vi "MC_7_12d_JW.vi"() -> ()   [LabVIEW 2011]
uses:
  <vilib>/Utility/file.llb/Read From Spreadsheet File (string).vi
  <vilib>/Utility/inputDevices.llb/keyboardAcquire.vi
  <vilib>/Utility/file.llb/Write To Spreadsheet File (DBL).vi
  <vilib>/Utility/file.llb/Write To Spreadsheet File (string).vi
  <vilib>/regexp/Match Regular Expression.xnode
panel:
  out "Rec: Temp":dbl
  out "Comments":string
  out "Folder Index":dbl caption="Length"
  out "Current \nRecord":string[](array[string])
  out "Transformer \nHeaders":string[](array[string])
  out "Current Device ID":string
  out "Column":string
  out "Row":string
  out "Rec: Concentration":dbl
  out "Rec: Solvent":string
  out "Rec: Method":string
  in  "?":T1(tab)
  out "Rec: Material":string
  in  "Treatment Concentration (mM):":dbl=30.0
  in  "Surface Treatment:":string
  in  "# Drops*:":dbl=inf
  in  "Solution Temp (C):":dbl=55.0
  in  "Relative Humidity (%):":dbl=nan
  in  "Room Temp (F):":dbl=nan
  in  "Time (s):":dbl=80.0
  out "Accel (RPM/s):":dbl
  in  "RPM:":dbl=1000.0
  in  "Wait Time (s):":dbl=10.0
  in  "Sample #:":dbl=1.0
  in  "Fabricator:":string="Jeremy"
  in  "Data File":path
  out "Data Folder":path
  in  "Image Folder":path
  out "Image File":path=path "D:/UserData/Desktop/Jeremy/WFU/Research/Programs/VI mods/Image Not Found.png"
  in  "Ramp (s):":dbl=3.0
  out "Calc: Trap Density-STS":dbl format="%#_4e"
  out "New: Trap Density-STS":dbl format="%#_4e"
  out "Rec: Trap Density-STS":dbl caption="Trap Density-STS" format="%#_3e"
  out "Calc: Trap Density-VT":dbl format="%#_4e"
  out "New: Trap Density-VT":dbl format="%#_4e"
  out "Rec: Trap Density-VT":dbl caption="Trap Density-VT" format="%#_3e"
  out "Calc: Onset V":dbl
  out "New: Onset":dbl
  out "Rec: Onset V":dbl caption="Onset V" format="%#_3g"
  out "Calc: Mobility-Lin":dbl format="%#_4e"
  out "New: Mobility-Lin":dbl format="%#_4e"
  out "Rec: Mobility-Lin":dbl caption="Mobility-Lin" format="%#_3e"
  out "Calc: Mobility-Sat":dbl format="%#_4e"
  out "Rec: Length":dbl caption="Length" format="%#_3g"
  out "Rec: Width":dbl caption="Width" format="%#_4g"
  out "Rec: Dielectric (d)":dbl caption="Dielectric (d)" format="%#_3g"
  out "XY Graph":cluster{dbl[], dbl[]}[](graph)
  in  "NumPts":dbl=5.0
  in  "Cancel Button":bool
  in  "Next Button":bool
  in  "Previous Button":bool
  in  "Up Button":bool
  in  "Down Button":bool
  out "Data Name:":string
  in  "Save Changes?":bool
  in  "New: Dielectric":dbl
  in  "New: Length":dbl
  in  "New: Width":dbl
  out "New: Mobility-Sat":dbl format="%#_4e"
  in  "Slide":dbl(slide) step=1.0 scale=-14.3..2.0 scale format="%#_1p"
  in  "Blank Button":bool
  in  "Zoom":i16(slide)=-3 scale=-5.0..5.0
  out "Image Out 2":T2(plugin-control)
  out "Image Out":T2(plugin-control)
  in  "Magnification":u16(ring) items=["5x", "10x", "20x", "50x", "80x"]
  out "Total Width":dbl
  out "Distances":dbl[](array[numeric])
  in  "Undo Button":bool
  in  "Remove Button":bool
  out "Rec: Mobility-Sat":dbl caption="Mobility-Sat" format="%#_3e"
  out "Index":string
  out "Image Name":string
  in  "Export":bool
  out "Calc: VT":dbl
  out "New: VT":dbl
  in  "Manual":bool
  out "XY Graph 2":cluster{dbl[], dbl[]}[](graph)
  in  "Next Button 2":bool
  in  "Previous Button 2":bool
  in  "Slide 2":dbl(slide) step=1.0 scale=-1.0..82.0 scale format="%#_1p"
  out "Calc: STS":dbl
  out "New: STS":dbl
  in  "NumPts 2":dbl=5.0 caption="NumPts"
  out "Rec: VT":dbl caption="Threshold V" format="%#_3g"
  out "Rec: STS":dbl caption="STS" format="%#_3g"
  out "Rec: On/Off":dbl caption="On/Off" format="%#_3e"
  in  "Save Changes? 2":bool
  in  "Save Changes? 3":bool
  out "Date Recorded":string="Date Recorded" caption="Recorded"
  out "Date Created":string caption="Fabricated"
  out "String":string
  in  "No Image":path=path "D:/UserData/Desktop/Jeremy/WFU/Research/Programs/VI mods/Image Not Found.png"
  in  "Project":path=path "D:/UserData/Desktop/Jeremy/WFU/Research/Programs/Mega Awesome/DeviceData.opj"
  out "Index 2":dbl
  out "Array 8":dbl[](array[numeric])
  out "Array 7":dbl[](array[numeric])
  out "ROI Descriptor out":T3 {"Contours"."Type" items=["No Selection", "Point", "Line", "Rectangle", "Oval", "Polygon", "Freehand Region", "Annulus", "Unused2", "Unused3", "Broken Line", "Freehand Line", "Rotated Rectangle"]}
  out "ROI Descriptor":T3 {"Contours"."Type" items=["No Selection", "Point", "Line", "Rectangle", "Oval", "Polygon", "Freehand Region", "Annulus", "Unused2", "Unused3", "Broken Line", "Freehand Line", "Rotated Rectangle"]}
  out "Numeric 3":dbl
  out "Array 6":dbl[][](array[numeric])
  out "Cluster":T4
  out "Array 5":dbl[](array[numeric])
  out "Array 4":dbl[](array[numeric])
  out "Array 3":dbl[](array[numeric])
  out "Numeric 2":dbl
  out "Numeric":dbl
  out "Array 2":dbl[](array[numeric])
  out "Array":dbl[](array[numeric])
  out "MobVi Index":dbl
  out "Table Control 2":string[][](table)
  out "Table Control":string[][](table)
  in  "Row Start":dbl=20.0
  # "Data Locations"
  # "Data Location"
  # "Image Location"
  # "Sample Properties"
  # "*     Inf = Full coverage\n   NaN = Unknown or Not Applicable"
  # "Recorded"
  # "Calculated"
  # "Re-Calculated"
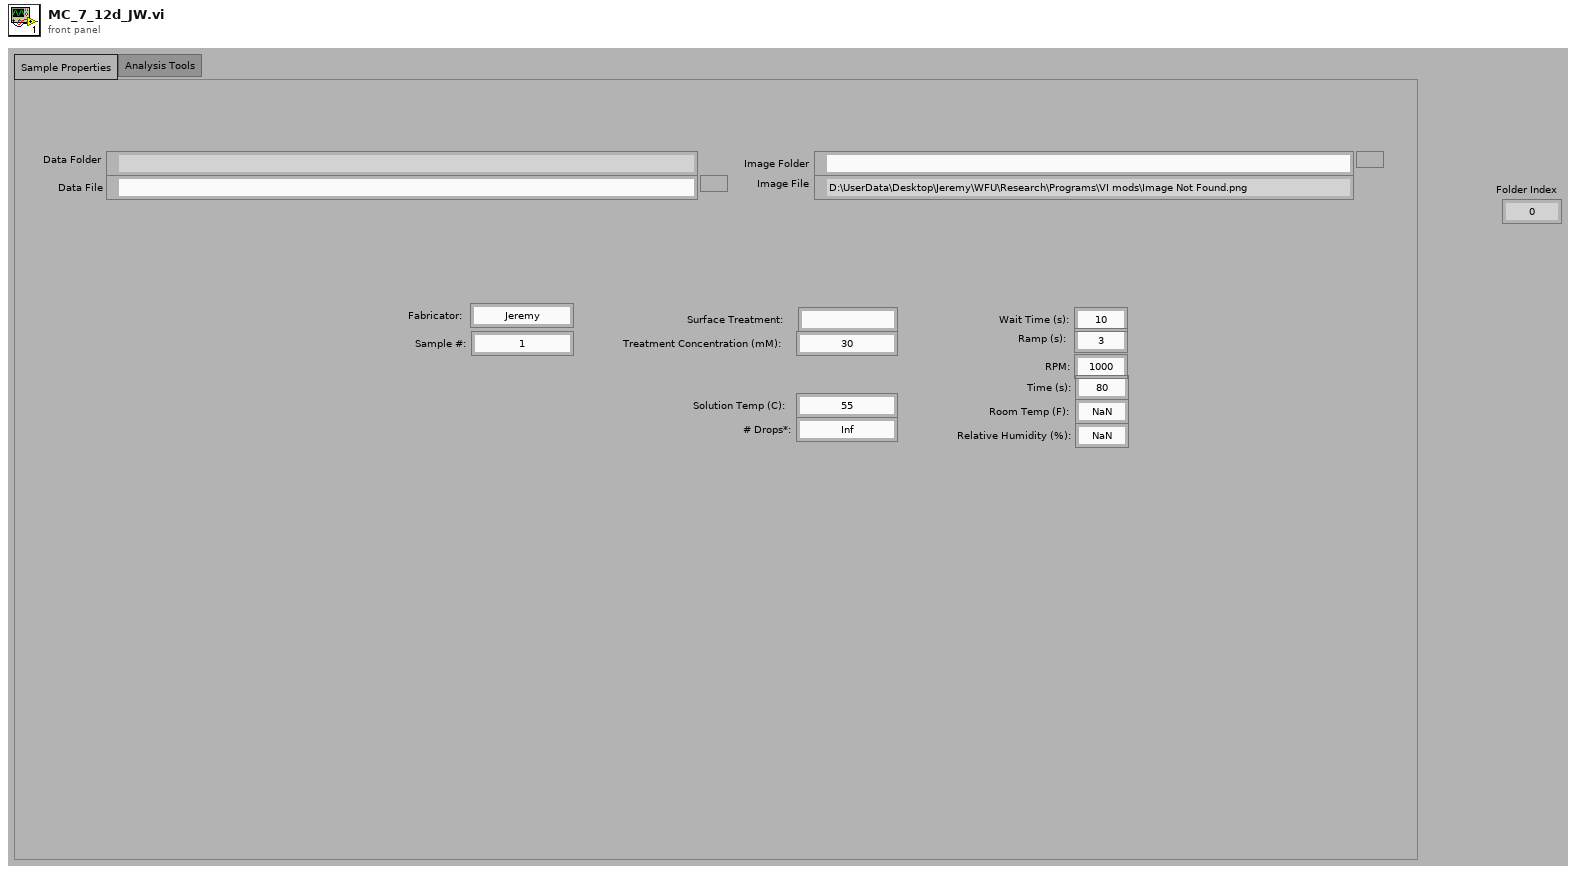
[diagram p1: front panel]
types:
  T1 = enum32{"Sample Properties", "Analysis Tools", "Current Database"}
  T2 = typedef "IMAQ Image.ctl" = refnum<image>
  T3 = typedef "ROI Descriptor" = cluster{"Global Rectangle":i32[], "Contours":cluster{"ID":enum32{"External", "Internal"}, "Type":u32, "Coordinates":i32[]}[]}
  T4 = cluster{"Numeric":dbl, "Numeric 2":dbl, "Numeric 3":dbl, "Numeric 4":dbl}
  T5 = cluster{"Mobility-Sat":dbl, "Moblitity-Lin":dbl, "On/Off":dbl, "Threshold Voltage":dbl, "Onset Voltage":dbl, "STS":dbl, "Trap Density-VT":dbl, "Trap Density-STS":dbl}
  T6 = cluster{"Date Recorded":string, "Index":string, "Length":dbl, "Width":dbl, "Sample Temp":dbl}
  T7 = cluster{"Date Created":string, "Material":string, "Solvent":string, "Concentration":dbl, "Method":string, "Dielectric (nm)":dbl, "Treatment":string, "Comments":string}
  T8 = cluster{"[0]":cluster{dbl[], dbl[]}, "[1]":cluster{dbl[], dbl[]}, "[2]":cluster{dbl[], dbl[]}, "[3]":cluster{dbl[], dbl[]}, "[4]":cluster{dbl[], dbl[]}, "[5]":cluster{dbl[], dbl[]}, "[6]":cluster{dbl[], dbl[]}, "[7]":cluster{dbl[], dbl[]}, "[8]":cluster{dbl[], dbl[]}}
  T9 = cluster{"Global Rectangle":i32[], "Contours":cluster{"Contour Type":u32, "ROI Type":u32, "Points":i32[]}[]}
  T10 = typedef "LVBoundsTypeDef.ctl" = cluster{"Width":u32, "Height":u32}
  T11 = enum16{"0", "1", "2", "3", "4", "5", "6", "7", "8", "9", "A", "B", "C", "D", "E", "F", "G", "H", "I", "J", "K", "L", "M", "N", "O", "P", "Q", "R", "S", "T", "U", "V", "W", "X", "Y", "Z", "F1", "F2", "F3", "F4", "F5", "F6", "F7", "F8", "F9", "F10", "F11", "F12", "F13", "F14", "F15", "ADD", "BACK", "BACKSLASH", "CAPITAL", "COMMA", "DECIMAL", "DELETE", "DIVIDE", "DOWN", "END", "EQUALS", "ESCAPE", "GRAVE (`)", "HOME", "INSERT", "LBRACKET", "LCONTROL", "LEFT", "L ALT", "LSHIFT", "LWIN", "MINUS", "MULTIPLY", "NEXT", "NUMLOCK", "NUMPAD_0", "NUMPAD_1", "NUMPAD_2", "NUMPAD_3", "NUMPAD_4", "NUMPAD_5", "NUMPAD_6", "NUMPAD_7", "NUMPAD_8", "NUMPAD_9", "PAUSE", "PERIOD", "PRIOR (PG UP)", "RBRACKET", "RCONTROL", "RETURN", "RIGHT", "R ALT", "RSHIFT", "RWIN", "SCROLL", "SEMICOLON", "SLASH", "SPACE", "SUBTRACT", "TAB", "UP", "ENTER (num pad)", "' (quote)"}[]
  T12 = cluster{"Contour Type":u32, "ROI Type":u32, "Points":i32[]}[]
  T13 = cluster{i32[], cluster{"Contour Type":u32, "ROI Type":u32, "Points":i32[]}[]}
  T14 = enum16{"0", "1", "2", "3", "4", "5", "6", "7", "8", "9", "A", "B", "C", "D", "E", "F", "G", "H", "I", "J", "K", "L", "M", "N", "O", "P", "Q", "R", "S", "T", "U", "V", "W", "X", "Y", "Z", "F1", "F2", "F3", "F4", "F5", "F6", "F7", "F8", "F9", "F10", "F11", "F12", "F13", "F14", "F15", "ADD", "BACK", "BACKSLASH", "CAPITAL", "COMMA", "DECIMAL", "DELETE", "DIVIDE", "DOWN", "END", "EQUALS", "ESCAPE", "GRAVE (`)", "HOME", "INSERT", "LBRACKET", "LCONTROL", "LEFT", "L ALT", "LSHIFT", "LWIN", "MINUS", "MULTIPLY", "NEXT", "NUMLOCK", "NUMPAD_0", "NUMPAD_1", "NUMPAD_2", "NUMPAD_3", "NUMPAD_4", "NUMPAD_5", "NUMPAD_6", "NUMPAD_7", "NUMPAD_8", "NUMPAD_9", "PAUSE", "PERIOD", "PRIOR (PG UP)", "RBRACKET", "RCONTROL", "RETURN", "RIGHT", "R ALT", "RSHIFT", "RWIN", "SCROLL", "SEMICOLON", "SLASH", "SPACE", "SUBTRACT", "TAB", "UP", "ENTER (num pad)", "' (quote)"}
  T15 = cluster{string, sgl, bool, bool, bool, bool, bool, bool, i32}
  T16 = cluster{i32, cluster{string, sgl, bool, bool, bool, bool, bool, bool, i32}, i32, i32}
  T17 = cluster{"Contour Type":u32, "ROI Type":u32, "Points":i32[]}
  T18 = cluster{"Points[0]":i32, "Points[1]":i32, "Points[2]":i32, "Points[3]":i32, "Points[4]":i32, "Points[5]":i32, "Points[6]":i32, "Points[7]":i32, "Points[8]":i32}
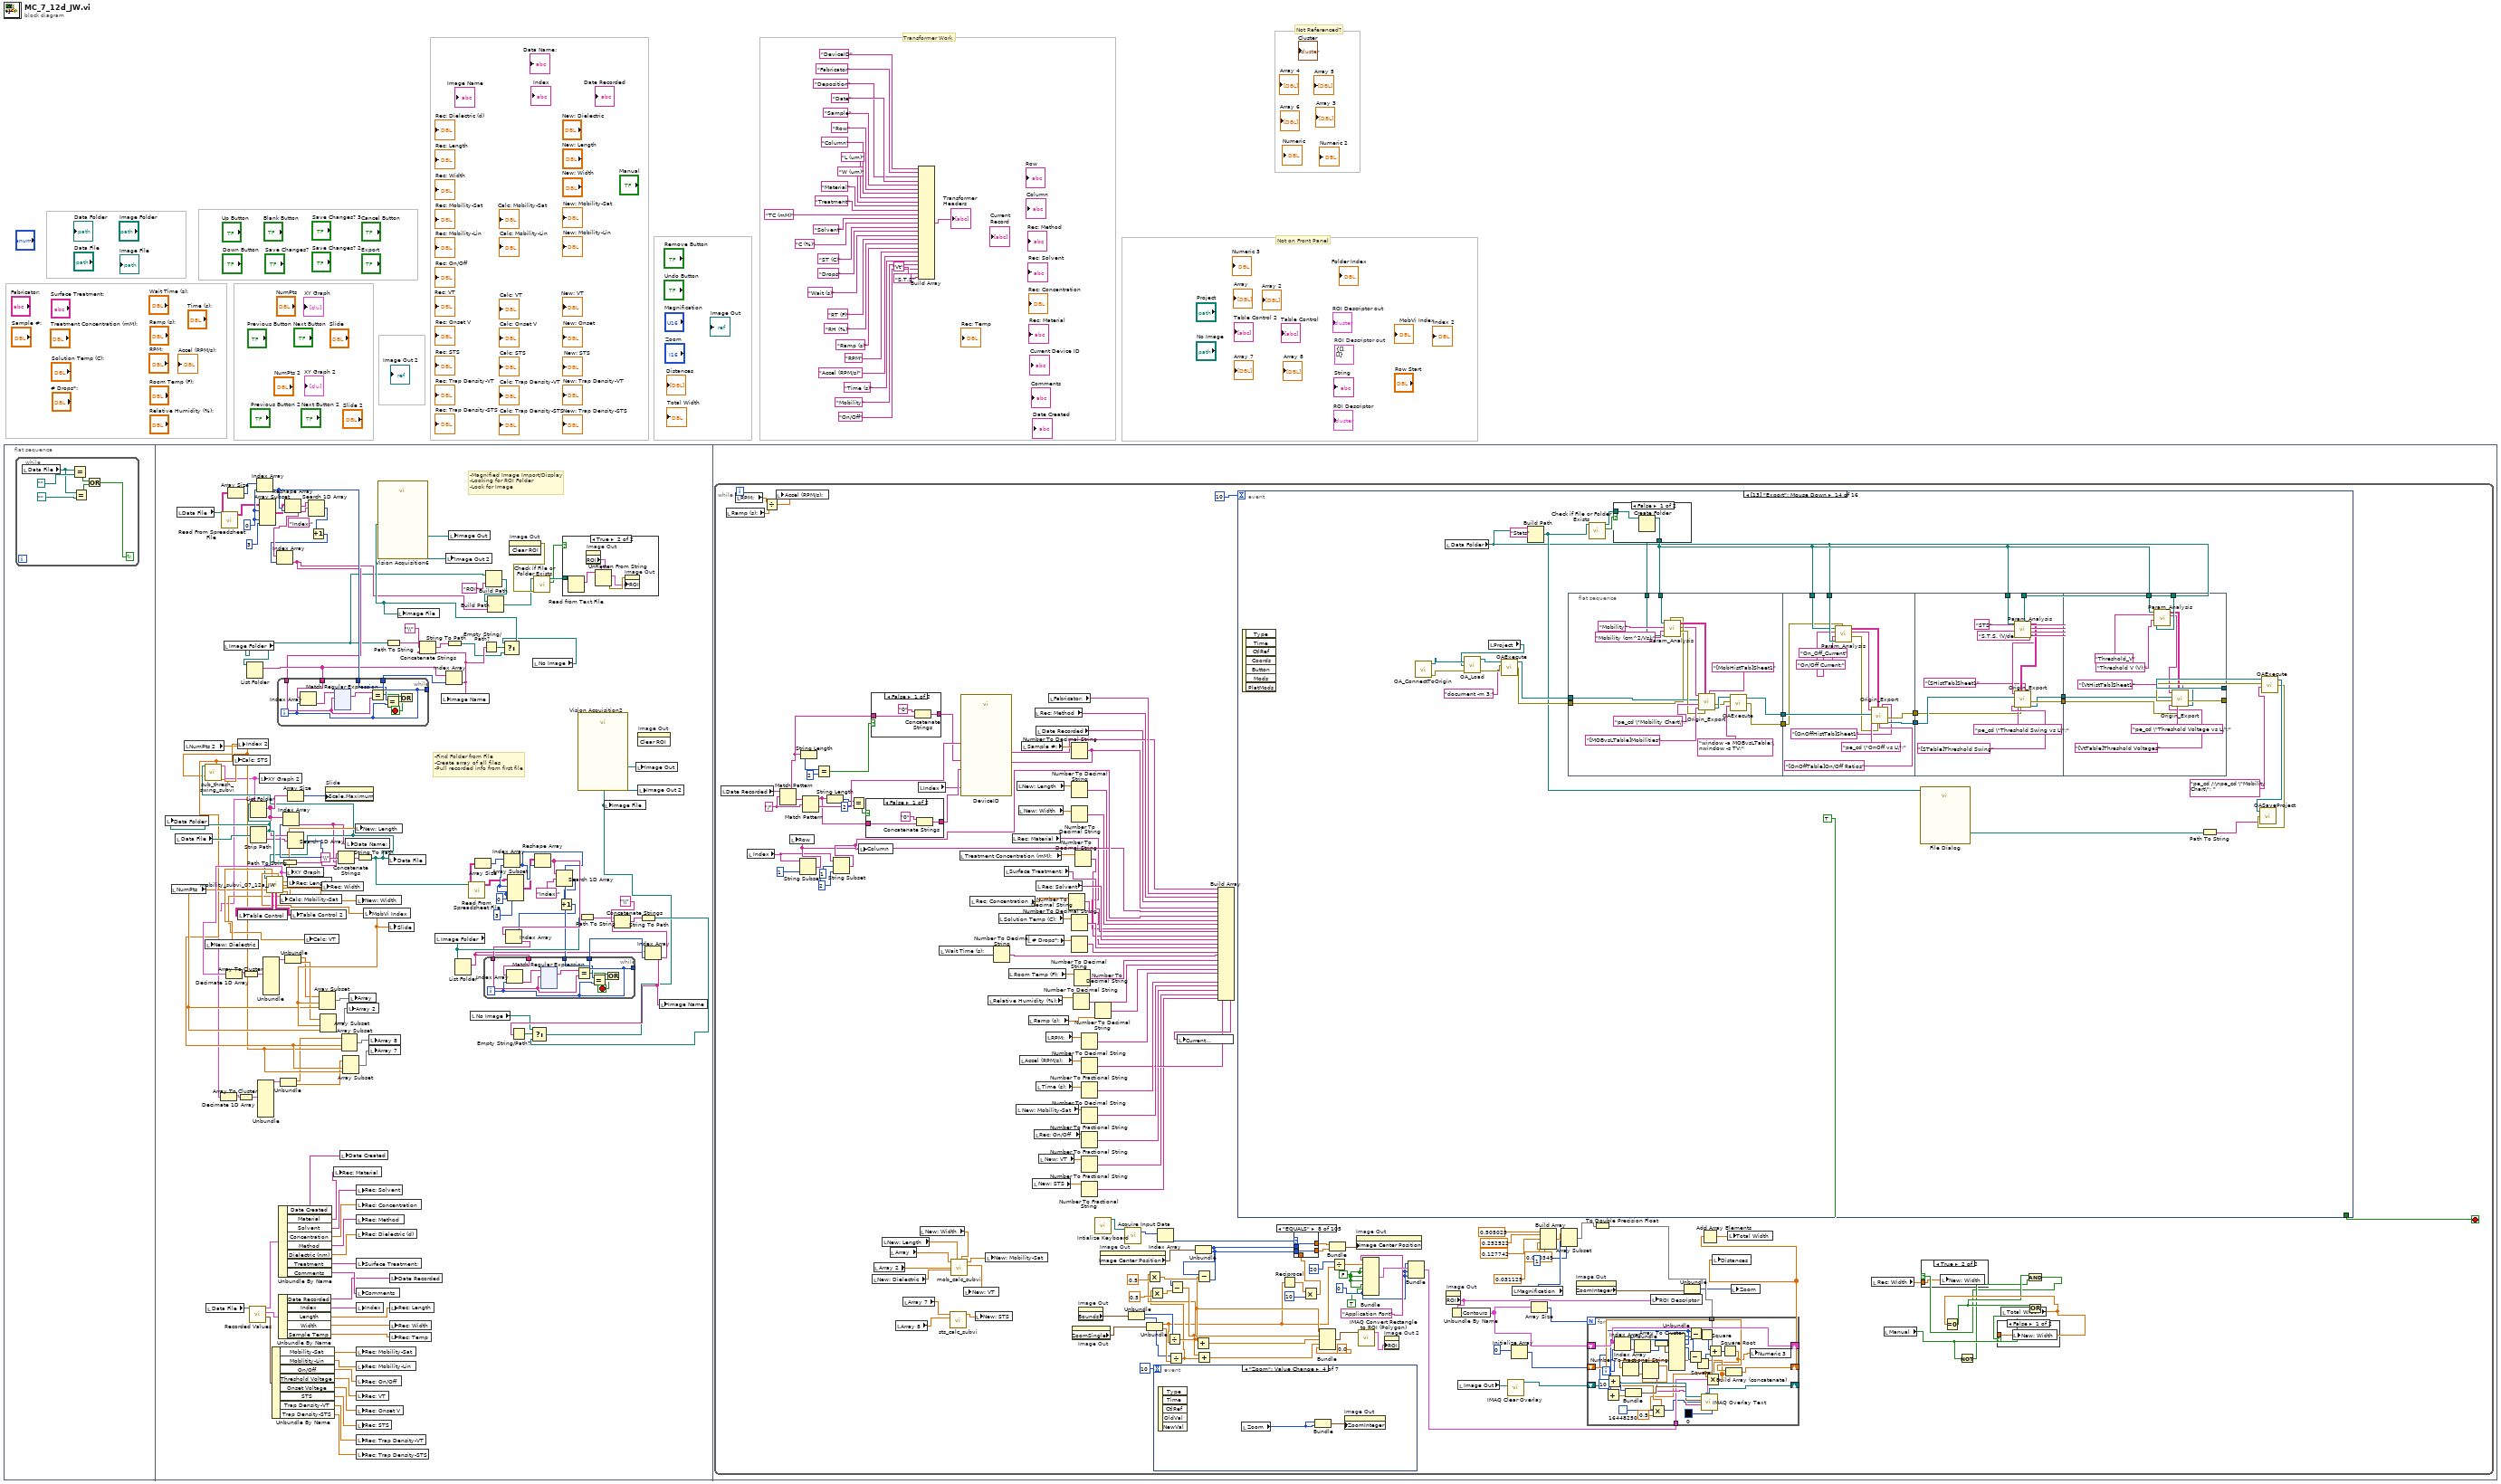
[diagram p0: block diagram]
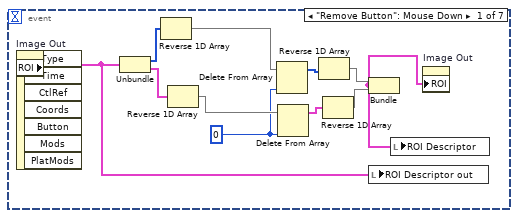
[diagram p7: hidden frame]
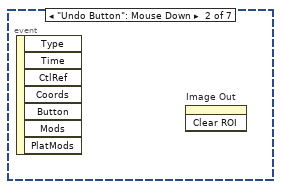
[diagram p8: hidden frame]
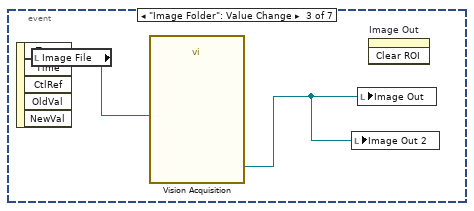
[diagram p9: hidden frame]
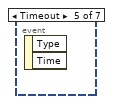
[diagram p10: hidden frame]
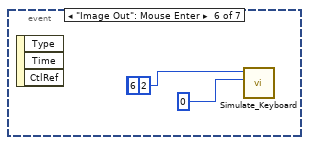
[diagram p11: hidden frame]
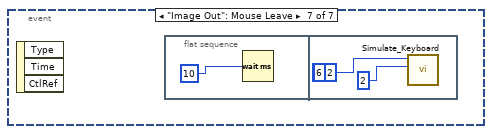
[diagram p12: hidden frame]
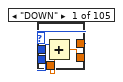
[diagram p13: hidden frame]
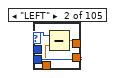
[diagram p14: hidden frame]
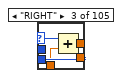
[diagram p15: hidden frame]
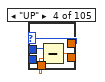
[diagram p16: hidden frame]
diagram:
  (unwired) T3 {"Global Rectangle"=[], "Contours"=[]}  # ROI Descriptor out
  # "Not Referenced?"
  # "Transformer Work"
  # "Not on Front Panel"
  n1 = flat-sequence {
    frame #0 {
      n2 = while {
        stop <- w29 continue-if-true
        n3 = local read "Data File"() -> (w31:path)
        n4 = Equal?(x=w31, y=path "") -> (x = y?=w33:bool)
        n5 = Equal?(x=w31, y=path "") -> (x = y?=w32:bool)
        n6 = Or(x=w33, y=w32) -> (x .or. y?=w29:bool)
      }
    }
    frame #1 {
      w115 = 0
      w140 = 0
      # "-Find Folder from File\n-Create array of all files\n-Pull recorded info from first file"
      # "-Magnified Image Import/Display\n-Looking for ROI Folder\n-Look for Image"
      n7 = local read "NumPts"() -> (w91:dbl)
      n8 = local read "Data File"() -> (w119:path)
      n9 = local read "Data File"() -> (w135:path)
      n10 = local read "NumPts 2"() -> (w86:dbl)
      n11 = local read "Data File"() -> (w59:path)
      n12 = call-poly <vilib>:"Read From Spreadsheet File.vi"("file path (dialog if empty)"=w135) -> ("all rows"=w138:string[][])  [unwired: 6 in, 4 out]
      n13 = local read "Image Folder"() -> (w61:path)
      n14 = Array Size(array=w138) -> (size(s)=w139:i32[])
      n15 = List Folder(path=w61) -> (filenames=w144:string[])  [unwired: 3 in, 3 out]
      n16 = call "Recorded Values.vi"("Path"=w59) -> ("Recorded Char"=w57:T5, "Recorded Prop"=w56:T6, "Fabrication Prop"=w58:T7)  [unwired: 8 in]
      n17 = Strip Path(path=w119) -> (stripped path=w120:path, name=w102:string)
      n18 = local write "Data Folder"(w120) -> ()
      n19 = List Folder(path=w120) -> (filenames=w109:string[])  [unwired: 3 in, 3 out]
      n20 = Index Array(array=w139, index=w140) -> (element=w146:i32)
      n21 = Array Subset(array=w138, index (row)=w140, index (col)=w140, length (col)=3) -> (w137:string[][])  [unwired: 1 in]
      n22 = Unbundle By Name(w57) -> ("Mobility-Sat"=w43:dbl, "Moblitity-Lin"=w42:dbl, "On/Off"=w41:dbl, "Threshold Voltage"=w40:dbl, "Onset Voltage"=w39:dbl, "STS"=w38:dbl, "Trap Density-VT"=w37:dbl, "Trap Density-STS"=w36:dbl)
      n23 = Unbundle By Name(w58) -> ("Date Created"=w35:string, "Material"=w55:string, "Solvent"=w54:string, "Concentration"=w53:dbl, "Method"=w52:string, "Dielectric (nm)"=w51:dbl, "Treatment"=w50:string, "Comments"=w49:string)
      n24 = Unbundle By Name(w56) -> ("Date Recorded"=w48:string, "Index"=w47:string, "Length"=w46:dbl, "Width"=w45:dbl, "Sample Temp"=w44:dbl)
      n25 = Path To String(path=w120) -> (string=w101:string)
      n26 = Reshape Array(w137, w146) -> (w151:string[])
      n27 = Array Size(array=w109) -> (size(s)=w110:i32)
      n28 = Search 1D Array(1D array=w109, element=w102) -> (index of element=w108:i32)  [unwired: 1 in]
      n29 = Index Array(array=w109, index=w108) -> (element=w60:string)
      n30 = Search 1D Array(1D array=w151, element="Index:") -> (index of element=w143:i32)  [unwired: 1 in]
      n31 = Increment(x=w143) -> (x+1=w142:i32)
      n32 = Index Array(array=w151, index=w142) -> (element=w62:string)
      n33 = while {
        tunnel: w144 -> [w284]
        tunnel: w62 -> [w282]
        tunnel: [w281] -> _
        tunnel: [w281] -> w145
        tunnel: w146 -> [w280]
        i -> [w281]
        stop <- w277 stop-if-true
        n34 = Index Array(array=w284, index=w281) -> (element=w285:string)
        n35 = xnode "Match Regular Expression"("input string"=w285, "regular expression"=w282) -> ("whole match"=w283:string)  [unwired: 4 in, 4 out]
        n36 = Equal?(x=w283, y=w282) -> (x = y?=w279:bool)
        n37 = Equal?(x=w280, y=w281) -> (x = y?=w278:bool)
        n38 = Or(x=w279, y=w278) -> (x .or. y?=w277:bool)
      }
      n39 = property on="Slide" class="Slide (strict)"("Scale.Maximum"=w110) -> ()  [unwired: 2 in, 2 out]
      n40 = local write "Rec: Material"(w55) -> ()
      n41 = Concatenate Strings(w101, "\\", w60) -> (w103:string)
      n42 = local write "Date Created"(w35) -> ()
      n43 = local write "Data Name:"(w60) -> ()
      n44 = local write "Rec: Solvent"(w54) -> ()
      n45 = local write "Rec: Concentration"(w53) -> ()
      n46 = local write "Rec: Method"(w52) -> ()
      n47 = local write "Rec: Dielectric (d)"(w51) -> ()
      n48 = local write "Surface Treatment:"(w50) -> ()
      n49 = local write "Comments"(w49) -> ()
      n50 = local write "Index"(w47) -> ()
      n51 = local write "Rec: Mobility-Sat"(w43) -> ()
      n52 = local write "Rec: Mobility-Lin"(w42) -> ()
      n53 = local write "Rec: On/Off"(w41) -> ()
      n54 = local write "Rec: VT"(w40) -> ()
      n55 = local write "Rec: Onset V"(w39) -> ()
      n56 = local write "Rec: STS"(w38) -> ()
      n57 = local write "Rec: Trap Density-VT"(w37) -> ()
      n58 = local write "Rec: Trap Density-STS"(w36) -> ()
      n59 = String To Path(string=w103) -> (path=w92:path)
      n60 = call "sub_thresh_swing_subvi.vi"("Path"=w92, "NumPts"=w86) -> ("Index"=w87:dbl, "XY Graph"=w82:cluster{dbl[], dbl[]}[], "Sub Threshold Swing"=w93:dbl)  [unwired: 9 in, 2 out]
      n61 = Decimate 1D Array(w82) -> (w83:cluster{dbl[], dbl[]}[])  [unwired: 1 out]
      n62 = local write "Calc: STS"(w93) -> ()
      n63 = local write "Index 2"(w87) -> ()
      n64 = Array To Cluster(array=w83) -> (cluster=w85:T8)
      n65 = Unbundle(w85) -> ("[0]"=w84:cluster{dbl[], dbl[]})  [unwired: 8 out]
      n66 = local write "XY Graph 2"(w82) -> ()
      n67 = call "mobility_subvi_07_12a_JW.vi"("Path"=w92, "NumPts"=w91) -> ("Dielectric (d)"=w97:dbl, "Index"=w98:dbl, "XY Graph"=w134:cluster{dbl[], dbl[]}[], "Length"=w96:dbl, "Vt"=w94:dbl, "Width"=w95:dbl, "Table Control"=w105:string[][], "Table Control 2"=w106:string[][], "Mobility"=w107:dbl)  [unwired: 4 in, 1 out]
      n68 = local write "New: Dielectric"(w97) -> ()
      n69 = Decimate 1D Array(w134) -> (w133:cluster{dbl[], dbl[]}[])  [unwired: 1 out]
      n70 = local write "Table Control"(w105) -> ()
      n71 = Array To Cluster(array=w133) -> (cluster=w131:T8)
      n72 = Unbundle(w131) -> ("[0]"=w132:cluster{dbl[], dbl[]})  [unwired: 8 out]
      n73 = local write "Calc: Mobility-Sat"(w107) -> ()
      n74 = Unbundle(w84) -> (w80:dbl[], w79:dbl[])
      n75 = Unbundle(w132) -> (w81:dbl[], w88:dbl[])
      n76 = local write "XY Graph"(w134) -> ()
      n77 = local write "Rec: Length"(w96) -> ()
      n78 = local write "Table Control 2"(w106) -> ()
      n79 = local write "Calc: VT"(w94) -> ()
      n80 = Array Subset(array=w81, index=w98, length=w91) -> (w99:dbl[])
      n81 = Array Subset(array=w88, index=w98, length=w91) -> (w100:dbl[])
      n82 = local write "Rec: Width"(w95) -> ()
      n83 = Array Subset(array=w80, index=w87, length=w86) -> (w90:dbl[])
      n84 = Array Subset(array=w79, index=w87, length=w86) -> (w89:dbl[])
      n85 = local write "Array 2"(w100) -> ()
      n86 = local write "Array"(w99) -> ()
      n87 = local write "New: Length"(w96) -> ()
      n88 = local write "New: Width"(w95) -> ()
      n89 = local write "MobVi Index"(w98) -> ()
      n90 = local write "Array 8"(w90) -> ()
      n91 = local write "Array 7"(w89) -> ()
      n92 = Path To String(path=w61) -> (string=w148:string)
      n93 = local write "Data File"(w92) -> ()
      n94 = local write "Slide"(w98) -> ()
      n95 = local write "Date Recorded"(w48) -> ()
      n96 = local write "Rec: Length"(w46) -> ()
      n97 = local write "Rec: Width"(w45) -> ()
      n98 = local write "Rec: Temp"(w44) -> ()
      n99 = local read "Image Folder"() -> (w126:path)
      n100 = Index Array(array=w144, index=w145) -> (element=w78:string)
      n101 = Concatenate Strings(w148, "\\", w78) -> (w149:string)
      n102 = local write "Image Name"(w78) -> ()
      n103 = String To Path(string=w149) -> (path=w76:path)
      n104 = List Folder(path=w126) -> (filenames=w122:string[])  [unwired: 3 in, 3 out]
      n105 = call-poly <vilib>:"Read From Spreadsheet File.vi"("file path (dialog if empty)"=w92) -> ("all rows"=w113:string[][])  [unwired: 6 in, 4 out]
      n106 = local read "No Image"() -> (w70:path)
      n107 = Array Size(array=w113) -> (size(s)=w114:i32[])
      n108 = Empty String/Path?(string/path=w78) -> (empty?=w77:bool)
      n109 = Build Path(base path=w61, name or relative path="ROI") -> (appended path=w64:path)
      n110 = Build Path(base path=w64, name or relative path=w62) -> (appended path=w63:path)
      n111 = Index Array(array=w114, index=w115) -> (element=w125:i32)
      n112 = Array Subset(array=w113, index (row)=w115, index (col)=w115, length (col)=3) -> (w112:string[][])  [unwired: 1 in]
      n113 = invoke on="Image Out" class="ImageControl" method="Clear ROI"() -> (error out=w68:errorcluster)  [unwired: 3 in, 2 out]
      n114 = local read "No Image"() -> (w69:path)
      n115 = Select(t=w69, s=w77, f=w76) -> (s? t:f=w75:path)
      n116 = call "Vision Acquisition6"("Image Path"=w75) -> ("Image Out"=w147:T2)  [unwired: 25 in, 1 out]
      n117 = local write "Image File"(w75) -> ()
      n118 = local write "Image Out 2"(w147) -> ()
      n119 = local write "Image Out"(w147) -> ()
      n120 = call <vilib>:"Check if File or Folder Exists.vi"("error in (no error)"=w68, "path"=w63) -> ("file or folder exists?"=w66:bool, "dup path"=w67:path)  [unwired: 7 in, 1 out]
      n121 = Reshape Array(w112, w125) -> (w130:string[])
      n122 = Search 1D Array(1D array=w130, element="Index:") -> (index of element=w118:i32)  [unwired: 1 in]
      n123 = Increment(x=w118) -> (x+1=w117:i32)
      n124 = Index Array(array=w130, index=w117) -> (element=w123:string)
      n125 = while {
        tunnel: w122 -> [w164]
        tunnel: w123 -> [w162]
        tunnel: [w161] -> _
        tunnel: [w161] -> w124
        tunnel: w125 -> [w160]
        i -> [w161]
        stop <- w157 stop-if-true
        n126 = Index Array(array=w164, index=w161) -> (element=w165:string)
        n127 = xnode "Match Regular Expression"("input string"=w165, "regular expression"=w162) -> ("whole match"=w163:string)  [unwired: 4 in, 4 out]
        n128 = Equal?(x=w163, y=w162) -> (x = y?=w159:bool)
        n129 = Equal?(x=w160, y=w161) -> (x = y?=w158:bool)
        n130 = Or(x=w159, y=w158) -> (x .or. y?=w157:bool)
      }
      n131 = case shown="True" w66 {
        tunnel: w67 -> [_ w152]
        frame False {
        }
        frame True {
          n132 = Read from Text File(file (use dialog)=w152) -> (text=w156:string)  [unwired: 3 in, 3 out]
          n133 = property on="Image Out" class="ImageControl"() -> ("ROI"=w153:T9)  [unwired: 2 in, 2 out]
          n134 = Unflatten From String(type=w153, binary string=w156) -> (value=w154:T9, error out=w155:errorcluster)  [unwired: 3 in, 1 out]
          n135 = property on="Image Out" class="ImageControl"(error in=w155, "ROI"=w154) -> ()  [unwired: 1 in, 2 out]
        }
      }
      n136 = Path To String(path=w126) -> (string=w127:string)
      n137 = invoke on="Image Out" class="ImageControl" method="Clear ROI"() -> ()  [unwired: 3 in, 3 out]
      n138 = Index Array(array=w122, index=w124) -> (element=w73:string)
      n139 = Empty String/Path?(string/path=w73) -> (empty?=w74:bool)
      n140 = Concatenate Strings(w127, "\\", w73) -> (w128:string)
      n141 = String To Path(string=w128) -> (path=w72:path)
      n142 = Select(t=w70, s=w74, f=w72) -> (s? t:f=w71:path)
      n143 = call "Vision Acquisition2"("Image Path"=w71) -> ("Image Out"=w121:T2)  [unwired: 25 in, 1 out]
      n144 = local write "Image File"(w71) -> ()
      n145 = local write "Image Out"(w121) -> ()
      n146 = local write "Image Out 2"(w121) -> ()
      n147 = local write "Image Name"(w73) -> ()
    }
    frame #2 {
      n148 = while {
        stop <- w544 stop-if-true
        w430 = "/"
        w494 = FALSE
        w492 = 0
        n149 = local read "Date Recorded"() -> (w433:string)
        n150 = local read "Ramp (s):"() -> (w400:dbl)
        n151 = local read "RPM:"() -> (w401:dbl)
        n152 = local read "Index"() -> (w403:string)
        n153 = Divide(x=w401, y=w400) -> (x/y=w399:dbl)
        n154 = local write "Accel (RPM/s):"(w399) -> ()
        n155 = Match Pattern(string=w433, regular expression=w430) -> (before substring=w424:string, after substring=w431:string)  [unwired: 1 in, 2 out]
        n156 = String Subset(string=w403, length (rest)=1) -> (substring=w458:string)  [unwired: 1 in]
        n157 = local write "Row"(w458) -> ()
        n158 = String Length(string=w424) -> (length=w427:i32)
        n159 = Match Pattern(string=w431, regular expression=w430) -> (before substring=w418:string, after substring=w429:string)  [unwired: 1 in, 2 out]
        n160 = Equal?(x=w427, y=2) -> (x = y?=w425:bool)
        n161 = String Length(string=w418) -> (length=w420:i32)
        n162 = String Subset(string=w403, offset (0)=1, length (rest)=2) -> (substring=w459:string)
        n163 = Equal?(x=w420, y=2) -> (x = y?=w422:bool)
        n164 = local write "Column"(w459) -> ()
        n165 = case shown="False" w422 {
          tunnel: w418 -> [w546 w548]
          tunnel: [w545 w548] -> w419
          frame False {
            n166 = Concatenate Strings("0", w546) -> (w545:string)
          }
          frame True {
          }
        }
        n167 = case shown="False" w425 {
          tunnel: w424 -> [w550 w552]
          tunnel: [w549 w552] -> w423
          frame False {
            n168 = Concatenate Strings("0", w550) -> (w549:string)
          }
          frame True {
          }
        }
        n169 = local read "New: Dielectric"() -> (w482:dbl)
        n170 = local read "Array 2"() -> (w478:dbl[])
        n171 = local read "New: Length"() -> (w480:dbl)
        n172 = local read "Array"() -> (w479:dbl[])
        n173 = local read "Array 8"() -> (w474:dbl[])
        n174 = local read "Array 7"() -> (w475:dbl[])
        n175 = local read "Index"() -> (w417:string)
        n176 = local read "New: Width"() -> (w483:dbl)
        n177 = local read "Wait Time (s):"() -> (w463:dbl)
        n178 = call "sts_calc_subvi.vi"("Array 2"=w474, "Array"=w475) -> ("STS"=w476:dbl)  [unwired: 9 in]
        n179 = call "mob_calc_subvi.vi"("Width"=w483, "Length"=w480, "Dielectric (d)"=w482, "Array 2"=w478, "Array"=w479) -> ("Vt"=w477:dbl, "Mobility"=w481:dbl)  [unwired: 4 in, 1 out]
        n180 = local read "Treatment Concentration (mM):"() -> (w411:dbl)
        n181 = local write "New: VT"(w477) -> ()
        n182 = local read "Rec: Concentration"() -> (w398:dbl)
        n183 = local write "New: STS"(w476) -> ()
        n184 = local write "New: Mobility-Sat"(w481) -> ()
        n185 = local read "Relative Humidity (%):"() -> (w408:dbl)
        n186 = Number To Decimal String(number=w463) -> (decimal integer string=w464:string)  [unwired: 1 in]
        n187 = local read "Solution Temp (C):"() -> (w452:dbl)
        n188 = local read "Surface Treatment:"() -> (w410:string)
        n189 = local read "Room Temp (F):"() -> (w456:dbl)
        n190 = local read "Rec: Material"() -> (w406:string)
        n191 = local read "New: Mobility-Sat"() -> (w445:dbl)
        n192 = local read "New: Length"() -> (w416:dbl)
        n193 = local read "New: Width"() -> (w415:dbl)
        n194 = local read "Accel (RPM/s):"() -> (w443:dbl)
        n195 = local read "Sample #:"() -> (w435:dbl)
        n196 = local read "# Drops*:"() -> (w453:dbl)
        n197 = local read "Ramp (s):"() -> (w461:dbl)
        n198 = local read "New: STS"() -> (w437:dbl)
        n199 = local read "Rec: On/Off"() -> (w441:dbl)
        n200 = local read "Rec: Method"() -> (w436:string)
        n201 = local read "Date Recorded"() -> (w432:string)
        n202 = local read "Rec: Solvent"() -> (w412:string)
        n203 = local read "Time (s):"() -> (w448:dbl)
        n204 = local read "New: VT"() -> (w439:dbl)
        n205 = local read "RPM:"() -> (w449:dbl)
        n206 = local read "Fabricator:"() -> (w457:string)
        n207 = Number To Decimal String(number=w398) -> (decimal integer string=w397:string)  [unwired: 1 in]
        n208 = Number To Decimal String(number=w453) -> (decimal integer string=w454:string)  [unwired: 1 in]
        n209 = Number To Decimal String(number=w435) -> (decimal integer string=w428:string)  [unwired: 1 in]
        n210 = call "DeviceID"("Sample"=w428, "Year"=w429, "Month"=w423, "Day"=w419, "Index"=w417) -> ("Result"=w434:string)  [unwired: 9 in, 1 out]
        n211 = Number To Decimal String(number=w416) -> (decimal integer string=w414:string)  [unwired: 1 in]
        n212 = Number To Decimal String(number=w415) -> (decimal integer string=w413:string)  [unwired: 1 in]
        n213 = Number To Decimal String(number=w452) -> (decimal integer string=w451:string)  [unwired: 1 in]
        n214 = property on="Image Out" class="ImageControl"() -> ("ZoomSingle"=w512:cluster{"X":sgl, "Y":sgl})  [unwired: 2 in, 2 out]
        n215 = Number To Decimal String(number=w408) -> (decimal integer string=w407:string)  [unwired: 1 in]
        n216 = Number To Decimal String(number=w456) -> (decimal integer string=w455:string)  [unwired: 1 in]
        n217 = Number To Decimal String(number=w411) -> (decimal integer string=w409:string)  [unwired: 1 in]
        n218 = property on="Image Out" class="ImageControl"() -> ("Bounds"=w513:T10)  [unwired: 2 in, 2 out]
        n219 = Number To Decimal String(number=w449) -> (decimal integer string=w450:string)  [unwired: 1 in]
        n220 = Number To Fractional String(number=w443) -> (F-format string=w444:string)  [unwired: 3 in]
        n221 = Number To Decimal String(number=w448) -> (decimal integer string=w447:string)  [unwired: 1 in]
        n222 = Number To Fractional String(number=w445) -> (F-format string=w446:string)  [unwired: 3 in]
        n223 = Number To Fractional String(number=w441) -> (F-format string=w442:string)  [unwired: 3 in]
        n224 = Number To Fractional String(number=w439) -> (F-format string=w440:string)  [unwired: 3 in]
        n225 = Number To Fractional String(number=w437) -> (F-format string=w438:string)  [unwired: 3 in]
        n226 = Number To Decimal String(number=w461) -> (decimal integer string=w462:string)  [unwired: 1 in]
        n227 = call <vilib>:"Intialize Keyboard.vi"() -> ("device ID"=w524:refnum<k1>)  [unwired: 10 in, 1 out]
        n228 = property on="Image Out" class="ImageControl"() -> ("Image Center Position"=w519:cluster{"X":u32, "Y":u32})  [unwired: 2 in, 2 out]
        n229 = call-poly <vilib>:"Acquire Input Data.vi"("device ID"=w524) -> ("keys pressed"=w523:T11)  [unwired: 16 in, 2 out]
        n230 = Unbundle(w513) -> ("Width"=w510:u32, "Height"=w509:u32)
        n231 = Unbundle(w512) -> ("X"=w487:sgl, "Y"=w511:sgl)
        n232 = event shown="[3] \"Zoom\": Value Change" {
          selector: _ -> [_ _ _ _ _ _ _]
          dyn-events: _ -> [_ _ _ _ _ _ _]
          timeout: 10 -> [_ _ _ _ _ _ _]
          event "Remove Button": Mouse Down {
            w557 = 0
            n233 = property on="Image Out" class="ImageControl"() -> ("ROI"=w555:T9)  [unwired: 2 in, 2 out]
            n234 = event-data() -> ()  [unwired: 1 in, 7 out]
            n235 = Unbundle(w555) -> ("Global Rectangle"=w558:i32[], "Contours"=w560:T12)
            n236 = Reverse 1D Array(array=w558) -> (reversed array=w559:i32[])
            n237 = Reverse 1D Array(array=w560) -> (reversed array=w561:T12)
            n238 = Delete From Array(array=w559, index=w557) -> (array with subset deleted=w562:i32[])  [unwired: 1 in, 1 out]
            n239 = Delete From Array(array=w561, index=w557) -> (array with subset deleted=w563:T12)  [unwired: 1 in, 1 out]
            n240 = Reverse 1D Array(array=w562) -> (reversed array=w564:i32[])
            n241 = Reverse 1D Array(array=w563) -> (reversed array=w565:T12)
            n242 = Bundle(w564, w565) -> (w556:T13)  [unwired: 1 in]
            n243 = local write "ROI Descriptor out"(w555) -> ()
            n244 = local write "ROI Descriptor"(w556) -> ()
            n245 = property on="Image Out" class="ImageControl"("ROI"=w556) -> ()  [unwired: 2 in, 2 out]
          }
          event "Undo Button": Mouse Down {
            n246 = event-data() -> ()  [unwired: 1 in, 7 out]
            n247 = invoke on="Image Out" class="ImageControl" method="Clear ROI"() -> ()  [unwired: 3 in, 3 out]
          }
          event "Image Folder": Value Change {
            n248 = event-data() -> ()  [unwired: 1 in, 5 out]
            n249 = local read "Image File"() -> (w567:path)
            n250 = call "Vision Acquisition"("Image Path"=w567) -> ("Image Out"=w566:T2)  [unwired: 25 in, 1 out]
            n251 = local write "Image Out 2"(w566) -> ()
            n252 = local write "Image Out"(w566) -> ()
            n253 = invoke on="Image Out" class="ImageControl" method="Clear ROI"() -> ()  [unwired: 3 in, 3 out]
          }
          event "Zoom": Value Change {
            n254 = event-data() -> ()  [unwired: 1 in, 5 out]
            n255 = local read "Zoom"() -> (w568:i16)
            n256 = Bundle("Zoom"=w568, "Zoom"=w568) -> (w569:cluster{"Zoom":i16, "Zoom":i16})  [unwired: 1 in]
            n257 = property on="Image Out" class="ImageControl"("ZoomInteger"=w569) -> ()  [unwired: 2 in, 2 out]
          }
          event Timeout {
            n258 = event-data() -> ()  [unwired: 1 in, 2 out]
          }
          event "Image Out": Mouse Enter {
            (unwired) 6
            n259 = event-data() -> ()  [unwired: 1 in, 3 out]
            n260 = call "Simulate_Keyboard.vi"("Action"=0, "Virtual Key"=162) -> ()  [unwired: 7 in, 1 out]
          }
          event "Image Out": Mouse Leave {
            n261 = event-data() -> ()  [unwired: 1 in, 3 out]
            n262 = flat-sequence {
              frame #0 {
                n263 = Wait (ms)(milliseconds to wait=10) -> ()  [unwired: 1 out]
              }
              frame #1 {
                (unwired) 6
                n264 = call "Simulate_Keyboard.vi"("Action"=2, "Virtual Key"=162) -> ()  [unwired: 7 in, 1 out]
              }
            }
          }
        }
        n265 = Index Array(array=w523) -> (element=w527:T14)  [unwired: 1 in]
        n266 = Divide(x=w510, y=w487) -> (x/y=w500:sgl)
        n267 = Multiply(x=w500, y=0.5) -> (x*y=w506:dbl)
        n268 = Divide(x=w509, y=w511) -> (x/y=w499:sgl)
        n269 = Multiply(x=w499, y=0.5) -> (x*y=w505:dbl)
        n270 = Unbundle(w519) -> ("X"=w501:u32, "Y"=w502:u32)
        n271 = Subtract(x=w502, y=w505) -> (x-y=w503:dbl)
        n272 = Subtract(x=w501, y=w506) -> (x-y=w504:dbl)
        n273 = Add(x=w504, y=w500) -> (x+y=w518:dbl)
        n274 = Add(x=w503, y=w499) -> (x+y=w517:dbl)
        n275 = Build Array(w434, w457, w436, w432, w428, w458, w459, w414, w413, w406, w410, w409, w412, w397, w451, w454, w464, w455, w407, w462, w450, w444, w447, w446, w442, w440, w438) -> (w460:string[])
        n276 = local write "Current \nRecord"(w460) -> ()
        n277 = event shown="[13] \"Export\": Mouse Down" {
          selector: _ -> [_ _ _ _ _ _ _ _ _ _ _ _ _ _ _ _]
          dyn-events: _ -> [_ _ _ _ _ _ _ _ _ _ _ _ _ _ _ _]
          timeout: 10 -> [_ _ _ _ _ _ _ _ _ _ _ _ _ _ _ _]
          tunnel: [_ _ _ _ _ _ _ _ _ _ _ _ _ TRUE _ TRUE] -> w544
          event Timeout {
            n278 = event-data() -> ()  [unwired: 1 in, 2 out]
          }
          event "Down Button": Mouse Down {
            w912 = 0
            n279 = event-data() -> ()  [unwired: 1 in, 7 out]
            n280 = local read "NumPts 2"() -> (w879:dbl)
            n281 = local read "NumPts"() -> (w885:dbl)
            n282 = local read "Folder Index"() -> (w851:dbl)
            n283 = local read "Data File"() -> (w917:path)
            n284 = local read "Data File"() -> (w849:path)
            n285 = call "Recorded Values.vi"("Path"=w849) -> ("Recorded Char"=w847:T5, "Recorded Prop"=w846:T6, "Fabrication Prop"=w848:T7)  [unwired: 8 in]
            n286 = Unbundle By Name(w847) -> ("Mobility-Sat"=w833:dbl, "Moblitity-Lin"=w832:dbl, "On/Off"=w831:dbl, "Threshold Voltage"=w830:dbl, "Onset Voltage"=w829:dbl, "STS"=w828:dbl, "Trap Density-VT"=w827:dbl, "Trap Density-STS"=w826:dbl)
            n287 = Unbundle By Name(w848) -> ("Date Created"=w825:string, "Material"=w845:string, "Solvent"=w844:string, "Concentration"=w843:dbl, "Method"=w842:string, "Dielectric (nm)"=w841:dbl, "Treatment"=w840:string, "Comments"=w839:string)
            n288 = Unbundle By Name(w846) -> ("Date Recorded"=w838:string, "Index"=w837:string, "Length"=w836:dbl, "Width"=w835:dbl, "Sample Temp"=w834:dbl)
            n289 = local write "Rec: Material"(w845) -> ()
            n290 = local write "Date Created"(w825) -> ()
            n291 = local write "Rec: Solvent"(w844) -> ()
            n292 = local write "Rec: Concentration"(w843) -> ()
            n293 = local write "Rec: Method"(w842) -> ()
            n294 = local write "Rec: Dielectric (d)"(w841) -> ()
            n295 = local write "Surface Treatment:"(w840) -> ()
            n296 = local write "Comments"(w839) -> ()
            n297 = local write "Index"(w837) -> ()
            n298 = local write "Rec: Mobility-Sat"(w833) -> ()
            n299 = local write "Rec: Mobility-Lin"(w832) -> ()
            n300 = local write "Rec: On/Off"(w831) -> ()
            n301 = local write "Rec: VT"(w830) -> ()
            n302 = local write "Rec: Onset V"(w829) -> ()
            n303 = local write "Rec: STS"(w828) -> ()
            n304 = local write "Rec: Trap Density-VT"(w827) -> ()
            n305 = local write "Rec: Trap Density-STS"(w826) -> ()
            n306 = property on="Image Out" class="ImageControl"() -> (error out=w852:errorcluster, "Image Center Position"=w856:cluster{"X":u32, "Y":u32})  [unwired: 2 in, 1 out]
            n307 = local write "Date Recorded"(w838) -> ()
            n308 = local write "Rec: Length"(w836) -> ()
            n309 = local write "Rec: Width"(w835) -> ()
            n310 = local write "Rec: Temp"(w834) -> ()
            n311 = Strip Path(path=w917) -> (stripped path=w908:path, name=w929:string)
            n312 = local write "Data Folder"(w908) -> ()
            n313 = List Folder(path=w908) -> (filenames=w922:string[], error out=w861:errorcluster)  [unwired: 3 in, 2 out]
            n314 = Array Size(array=w922) -> (size(s)=w918:i32)
            n315 = Path To String(path=w908) -> (string=w930:string)
            n316 = Search 1D Array(1D array=w922, element=w929) -> (index of element=w919:i32)  [unwired: 1 in]
            n317 = Unbundle(w856) -> ("X"=w854:u32)  [unwired: 1 out]
            n318 = Bundle("X"=w854, 0) -> (w855:cluster{"X":u32, i32})  [unwired: 1 in]
            n319 = Decrement(x=w918) -> (x-1=w920:i32)
            n320 = Equal?(x=w919, y=w920) -> (x = y?=w921:bool)
            n321 = case shown="False" w921 {
              tunnel: w851 -> [w1057 _]
              tunnel: [w1056 0] -> w850
              frame False {
                n322 = Increment(x=w1057) -> (x+1=w1056:dbl)
              }
              frame True {
              }
            }
            n323 = Index Array(array=w922, index=w850) -> (element=w923:string)
            n324 = local write "Folder Index"(w850) -> ()
            n325 = local write "Data Name:"(w923) -> ()
            n326 = Concatenate Strings(w930, "\\", w923) -> (w928:string)
            n327 = property on="Image Out" class="ImageControl"(error in=w852, "Image Center Position"=w855) -> ()  [unwired: 1 in, 2 out]
            n328 = String To Path(string=w928) -> (path=w886:path)
            n329 = call "sub_thresh_swing_subvi.vi"("Path"=w886, "NumPts"=w879) -> ("Index"=w880:dbl, "XY Graph"=w875:cluster{dbl[], dbl[]}[], "Sub Threshold Swing"=w887:dbl)  [unwired: 9 in, 2 out]
            n330 = Decimate 1D Array(w875) -> (w878:cluster{dbl[], dbl[]}[])  [unwired: 1 out]
            n331 = Array To Cluster(array=w878) -> (cluster=w876:T8)
            n332 = Unbundle(w876) -> ("[0]"=w877:cluster{dbl[], dbl[]})  [unwired: 8 out]
            n333 = Unbundle(w877) -> (w874:dbl[], w873:dbl[])
            n334 = local write "Calc: STS"(w887) -> ()
            n335 = local write "XY Graph 2"(w875) -> ()
            n336 = local write "Index 2"(w880) -> ()
            n337 = call "mobility_subvi_07_12a_JW.vi"("Path"=w886, "NumPts"=w885) -> ("Dielectric (d)"=w889:dbl, "Index"=w894:dbl, "XY Graph"=w897:cluster{dbl[], dbl[]}[], "Length"=w888:dbl, "Vt"=w890:dbl, "Width"=w867:dbl, "Table Control"=w926:string[][], "Table Control 2"=w925:string[][], "Mobility"=w924:dbl)  [unwired: 4 in, 1 out]
            n338 = local write "Calc: VT"(w890) -> ()
            n339 = local write "New: Dielectric"(w889) -> ()
            n340 = Decimate 1D Array(w897) -> (w898:cluster{dbl[], dbl[]}[])  [unwired: 1 out]
            n341 = Array To Cluster(array=w898) -> (cluster=w900:T8)
            n342 = local write "Table Control"(w926) -> ()
            n343 = Unbundle(w900) -> ("[0]"=w899:cluster{dbl[], dbl[]})  [unwired: 8 out]
            n344 = Unbundle(w899) -> (w882:dbl[], w881:dbl[])
            n345 = local write "Calc: Mobility-Sat"(w924) -> ()
            n346 = local write "XY Graph"(w897) -> ()
            n347 = local write "Table Control 2"(w925) -> ()
            n348 = Array Subset(array=w882, index=w894, length=w885) -> (w896:dbl[])
            n349 = Array Subset(array=w881, index=w894, length=w885) -> (w895:dbl[])
            n350 = local write "Array 2"(w895) -> ()
            n351 = local write "Array"(w896) -> ()
            n352 = local write "MobVi Index"(w894) -> ()
            n353 = local write "Slide"(w894) -> ()
            n354 = Array Subset(array=w874, index=w880, length=w879) -> (w884:dbl[])
            n355 = Array Subset(array=w873, index=w880, length=w879) -> (w883:dbl[])
            n356 = local write "New: Width"(w867) -> ()
            n357 = local write "Data File"(w886) -> ()
            n358 = local write "New: Length"(w888) -> ()
            n359 = local write "Array 8"(w884) -> ()
            n360 = local write "Array 7"(w883) -> ()
            n361 = call-poly <vilib>:"Read From Spreadsheet File.vi"("file path (dialog if empty)"=w886) -> ("all rows"=w914:string[][])  [unwired: 6 in, 4 out]
            n362 = local read "Image Folder"() -> (w858:path)
            n363 = Array Size(array=w914) -> (size(s)=w913:i32[])
            n364 = List Folder(path=w858, error in=w861) -> (filenames=w907:string[], error out=w862:errorcluster)  [unwired: 2 in, 2 out]
            n365 = Index Array(array=w913, index=w912) -> (element=w892:i32)
            n366 = Subtract(x=w892, y=20) -> (x-y=w891:i32)
            n367 = property on="Slide" class="Slide (strict)"("Scale.Maximum"=w891) -> ()  [unwired: 2 in, 2 out]
            n368 = Array Subset(array=w914, index (row)=w912, index (col)=w912, length (col)=3) -> (w915:string[][])  [unwired: 1 in]
            n369 = Reshape Array(w915, w892) -> (w901:string[])
            n370 = local read "No Image"() -> (w868:path)
            n371 = Search 1D Array(1D array=w901, element="Index:") -> (index of element=w909:i32)  [unwired: 1 in]
            n372 = Increment(x=w909) -> (x+1=w910:i32)
            n373 = Index Array(array=w901, index=w910) -> (element=w860:string)
            n374 = while {
              tunnel: w907 -> [w943]
              tunnel: w860 -> [w941]
              tunnel: [w940] -> _
              tunnel: [w940] -> w906
              tunnel: w892 -> [w939]
              i -> [w940]
              stop <- w936 stop-if-true
              n375 = Index Array(array=w943, index=w940) -> (element=w944:string)
              n376 = xnode "Match Regular Expression"("input string"=w944, "regular expression"=w941) -> ("whole match"=w942:string)  [unwired: 4 in, 4 out]
              n377 = Equal?(x=w942, y=w941) -> (x = y?=w938:bool)
              n378 = Equal?(x=w939, y=w940) -> (x = y?=w937:bool)
              n379 = Or(x=w938, y=w937) -> (x .or. y?=w936:bool)
            }
            n380 = Build Path(base path=w858, name or relative path="ROI") -> (appended path=w857:path)
            n381 = Build Path(base path=w857, name or relative path=w860) -> (appended path=w866:path)
            n382 = invoke on="Image Out" class="ImageControl" method="Clear ROI"(error in=w862) -> (error out=w865:errorcluster)  [unwired: 2 in, 2 out]
            n383 = Path To String(path=w858) -> (string=w904:string)
            n384 = invoke on="Image Out" class="ImageControl" method="Clear ROI"() -> ()  [unwired: 3 in, 3 out]
            n385 = call <vilib>:"Check if File or Folder Exists.vi"("error in (no error)"=w865, "path"=w866) -> ("file or folder exists?"=w863:bool, "dup path"=w864:path)  [unwired: 7 in, 1 out]
            n386 = case shown="True" w863 {
              tunnel: w864 -> [_ w931]
              frame False {
              }
              frame True {
                n387 = Read from Text File(file (use dialog)=w931) -> (text=w935:string)  [unwired: 3 in, 3 out]
                n388 = property on="Image Out" class="ImageControl"() -> ("ROI"=w932:T9)  [unwired: 2 in, 2 out]
                n389 = Unflatten From String(type=w932, binary string=w935) -> (value=w933:T9, error out=w934:errorcluster)  [unwired: 3 in, 1 out]
                n390 = property on="Image Out" class="ImageControl"(error in=w934, "ROI"=w933) -> ()  [unwired: 1 in, 2 out]
              }
            }
            n391 = Index Array(array=w907, index=w906) -> (element=w871:string)
            n392 = Empty String/Path?(string/path=w871) -> (empty?=w872:bool)
            n393 = Concatenate Strings(w904, "\\", w871) -> (w903:string)
            n394 = String To Path(string=w903) -> (path=w870:path)
            n395 = Select(t=w868, s=w872, f=w870) -> (s? t:f=w869:path)
            n396 = call "Vision Acquisition4"("Image Path"=w869) -> ("Image Out"=w905:T2)  [unwired: 25 in, 1 out]
            n397 = local write "Image File"(w869) -> ()
            n398 = local write "Image Out 2"(w905) -> ()
            n399 = local write "Image Out"(w905) -> ()
            n400 = local write "Image Name"(w871) -> ()
          }
          event "Data File": Value Change {
            w1151 = 0
            n401 = event-data() -> ()  [unwired: 1 in, 5 out]
            n402 = local read "Data File"() -> (w1083:path)
            n403 = call "Recorded Values.vi"("Path"=w1083) -> ("Recorded Char"=w1081:T5, "Recorded Prop"=w1080:T6, "Fabrication Prop"=w1082:T7)  [unwired: 8 in]
            n404 = Unbundle By Name(w1081) -> ("Mobility-Sat"=w1067:dbl, "Moblitity-Lin"=w1066:dbl, "On/Off"=w1065:dbl, "Threshold Voltage"=w1064:dbl, "Onset Voltage"=w1063:dbl, "STS"=w1062:dbl, "Trap Density-VT"=w1061:dbl, "Trap Density-STS"=w1060:dbl)
            n405 = Unbundle By Name(w1082) -> ("Date Created"=w1059:string, "Material"=w1079:string, "Solvent"=w1078:string, "Concentration"=w1077:dbl, "Method"=w1076:string, "Dielectric (nm)"=w1075:dbl, "Treatment"=w1074:string, "Comments"=w1073:string)
            n406 = Unbundle By Name(w1080) -> ("Date Recorded"=w1072:string, "Index"=w1071:string, "Length"=w1070:dbl, "Width"=w1069:dbl, "Sample Temp"=w1068:dbl)
            n407 = local write "Date Created"(w1059) -> ()
            n408 = local write "Rec: Material"(w1079) -> ()
            n409 = local read "NumPts"() -> (w1119:dbl)
            n410 = local read "Data File"() -> (w1147:path)
            n411 = local write "Rec: Solvent"(w1078) -> ()
            n412 = local write "Rec: Concentration"(w1077) -> ()
            n413 = local write "Rec: Method"(w1076) -> ()
            n414 = local write "Rec: Dielectric (d)"(w1075) -> ()
            n415 = local write "Surface Treatment:"(w1074) -> ()
            n416 = local write "Comments"(w1073) -> ()
            n417 = local write "Index"(w1071) -> ()
            n418 = local write "Rec: Mobility-Sat"(w1067) -> ()
            n419 = local write "Rec: Mobility-Lin"(w1066) -> ()
            n420 = local write "Rec: On/Off"(w1065) -> ()
            n421 = local write "Rec: VT"(w1064) -> ()
            n422 = local write "Rec: Onset V"(w1063) -> ()
            n423 = local write "Rec: STS"(w1062) -> ()
            n424 = local write "Rec: Trap Density-VT"(w1061) -> ()
            n425 = local write "Rec: Trap Density-STS"(w1060) -> ()
            n426 = local write "Date Recorded"(w1072) -> ()
            n427 = local write "Rec: Length"(w1070) -> ()
            n428 = local write "Rec: Width"(w1069) -> ()
            n429 = local write "Rec: Temp"(w1068) -> ()
            n430 = local read "NumPts 2"() -> (w1113:dbl)
            n431 = property on="Image Out" class="ImageControl"() -> (error out=w1085:errorcluster, "Image Center Position"=w1089:cluster{"X":u32, "Y":u32})  [unwired: 2 in, 1 out]
            n432 = Strip Path(path=w1147) -> (stripped path=w1146:path, name=w1163:string)
            n433 = local write "Data Folder"(w1146) -> ()
            n434 = List Folder(path=w1146) -> (filenames=w1156:string[], error out=w1095:errorcluster)  [unwired: 3 in, 2 out]
            n435 = Unbundle(w1089) -> ("X"=w1087:u32)  [unwired: 1 out]
            n436 = Path To String(path=w1146) -> (string=w1164:string)
            n437 = Search 1D Array(1D array=w1156, element=w1163) -> (index of element=w1084:i32)  [unwired: 1 in]
            n438 = Index Array(array=w1156, index=w1084) -> (element=w1157:string)
            n439 = Bundle("X"=w1087, 0) -> (w1088:cluster{"X":u32, i32})  [unwired: 1 in]
            n440 = local write "Data Name:"(w1157) -> ()
            n441 = property on="Image Out" class="ImageControl"(error in=w1085, "Image Center Position"=w1088) -> ()  [unwired: 1 in, 2 out]
            n442 = local write "Folder Index"(w1084) -> ()
            n443 = Concatenate Strings(w1164, "\\", w1157) -> (w1162:string)
            n444 = String To Path(string=w1162) -> (path=w1120:path)
            n445 = call "sub_thresh_swing_subvi.vi"("Path"=w1120, "NumPts"=w1113) -> ("Index"=w1114:dbl, "XY Graph"=w1109:cluster{dbl[], dbl[]}[], "Sub Threshold Swing"=w1118:dbl)  [unwired: 9 in, 2 out]
            n446 = Decimate 1D Array(w1109) -> (w1112:cluster{dbl[], dbl[]}[])  [unwired: 1 out]
            n447 = Array To Cluster(array=w1112) -> (cluster=w1110:T8)
            n448 = Unbundle(w1110) -> ("[0]"=w1111:cluster{dbl[], dbl[]})  [unwired: 8 out]
            n449 = Unbundle(w1111) -> (w1107:dbl[], w1106:dbl[])
            n450 = local write "Index 2"(w1114) -> ()
            n451 = call "mobility_subvi_07_12a_JW.vi"("Path"=w1120, "NumPts"=w1119) -> ("Dielectric (d)"=w1122:dbl, "Index"=w1127:dbl, "XY Graph"=w1130:cluster{dbl[], dbl[]}[], "Length"=w1121:dbl, "Vt"=w1123:dbl, "Width"=w1100:dbl, "Table Control"=w1160:string[][], "Table Control 2"=w1159:string[][], "Mobility"=w1158:dbl)  [unwired: 4 in, 1 out]
            n452 = local write "Rec: Dielectric (d)"(w1122) -> ()
            n453 = local write "New: Dielectric"(w1122) -> ()
            n454 = Decimate 1D Array(w1130) -> (w1131:cluster{dbl[], dbl[]}[])  [unwired: 1 out]
            n455 = local write "Table Control"(w1160) -> ()
            n456 = Array To Cluster(array=w1131) -> (cluster=w1133:T8)
            n457 = Unbundle(w1133) -> ("[0]"=w1132:cluster{dbl[], dbl[]})  [unwired: 8 out]
            n458 = local write "Calc: VT"(w1123) -> ()
            n459 = local write "Calc: STS"(w1118) -> ()
            n460 = local write "Calc: Mobility-Sat"(w1158) -> ()
            n461 = Unbundle(w1132) -> (w1108:dbl[], w1115:dbl[])
            n462 = local write "XY Graph"(w1130) -> ()
            n463 = local write "Table Control 2"(w1159) -> ()
            n464 = local write "XY Graph 2"(w1109) -> ()
            n465 = Array Subset(array=w1107, index=w1114, length=w1113) -> (w1117:dbl[])
            n466 = Array Subset(array=w1106, index=w1114, length=w1113) -> (w1116:dbl[])
            n467 = local write "New: Length"(w1121) -> ()
            n468 = local write "MobVi Index"(w1127) -> ()
            n469 = Array Subset(array=w1108, index=w1127, length=w1119) -> (w1129:dbl[])
            n470 = Array Subset(array=w1115, index=w1127, length=w1119) -> (w1128:dbl[])
            n471 = local write "Array 8"(w1117) -> ()
            n472 = local write "Array 7"(w1116) -> ()
            n473 = local write "New: Width"(w1100) -> ()
            n474 = local write "Array 2"(w1128) -> ()
            n475 = local write "Array"(w1129) -> ()
            n476 = local write "Data File"(w1120) -> ()
            n477 = local read "Image Folder"() -> (w1091:path)
            n478 = local write "Slide"(w1127) -> ()
            n479 = List Folder(path=w1091, error in=w1095) -> (filenames=w1144:string[], error out=w1094:errorcluster)  [unwired: 2 in, 2 out]
            n480 = call-poly <vilib>:"Read From Spreadsheet File.vi"("file path (dialog if empty)"=w1120) -> ("all rows"=w1153:string[][])  [unwired: 6 in, 4 out]
            n481 = Array Size(array=w1153) -> (size(s)=w1152:i32[])
            n482 = Index Array(array=w1152, index=w1151) -> (element=w1126:i32)
            n483 = Subtract(x=w1126, y=20) -> (x-y=w1124:i32)
            n484 = property on="Slide" class="Slide (strict)"("Scale.Maximum"=w1124) -> ()  [unwired: 2 in, 2 out]
            n485 = Array Subset(array=w1153, index (row)=w1151, index (col)=w1151, length (col)=3) -> (w1154:string[][])  [unwired: 1 in]
            n486 = Reshape Array(w1154, w1126) -> (w1134:string[])
            n487 = Search 1D Array(1D array=w1134, element="Index:") -> (index of element=w1148:i32)  [unwired: 1 in]
            n488 = Increment(x=w1148) -> (x+1=w1149:i32)
            n489 = Index Array(array=w1134, index=w1149) -> (element=w1093:string)
            n490 = while {
              tunnel: w1144 -> [w1177]
              tunnel: w1093 -> [w1175]
              tunnel: [w1174] -> _
              tunnel: [w1174] -> w1143
              tunnel: w1126 -> [w1173]
              i -> [w1174]
              stop <- w1170 stop-if-true
              n491 = Index Array(array=w1177, index=w1174) -> (element=w1178:string)
              n492 = xnode "Match Regular Expression"("input string"=w1178, "regular expression"=w1175) -> ("whole match"=w1176:string)  [unwired: 4 in, 4 out]
              n493 = Equal?(x=w1176, y=w1175) -> (x = y?=w1172:bool)
              n494 = Equal?(x=w1173, y=w1174) -> (x = y?=w1171:bool)
              n495 = Or(x=w1172, y=w1171) -> (x .or. y?=w1170:bool)
            }
            n496 = local write "Index"(w1093) -> ()
            n497 = Search 1D Array(1D array=w1134, element="Mobility-Sat (cm^2/Vs):") -> (index of element=w1139:i32)  [unwired: 1 in]
            n498 = Increment(x=w1139) -> (x+1=w1138:i32)
            n499 = Index Array(array=w1134, index=w1138) -> (element=w1136:string)
            n500 = Fract/Exp String To Number(string=w1136) -> (number=w1135:dbl)  [unwired: 3 in, 1 out]
            n501 = local write "Rec: Mobility-Sat"(w1135) -> ()
            n502 = Build Path(base path=w1091, name or relative path="ROI") -> (appended path=w1090:path)
            n503 = Path To String(path=w1091) -> (string=w1142:string)
            n504 = local read "No Image"() -> (w1101:path)
            n505 = Build Path(base path=w1090, name or relative path=w1093) -> (appended path=w1099:path)
            n506 = invoke on="Image Out" class="ImageControl" method="Clear ROI"(error in=w1094) -> (error out=w1098:errorcluster)  [unwired: 2 in, 2 out]
            n507 = Index Array(array=w1144, index=w1143) -> (element=w1104:string)
            n508 = Empty String/Path?(string/path=w1104) -> (empty?=w1105:bool)
            n509 = Concatenate Strings(w1142, "\\", w1104) -> (w1141:string)
            n510 = String To Path(string=w1141) -> (path=w1103:path)
            n511 = Select(t=w1101, s=w1105, f=w1103) -> (s? t:f=w1102:path)
            n512 = call "Vision Acquisition3"("Image Path"=w1102) -> ("Image Out"=w1145:T2)  [unwired: 25 in, 1 out]
            n513 = local write "Image File"(w1102) -> ()
            n514 = local write "Image Out 2"(w1145) -> ()
            n515 = local write "Image Out"(w1145) -> ()
            n516 = local write "Image Name"(w1104) -> ()
            n517 = call <vilib>:"Check if File or Folder Exists.vi"("error in (no error)"=w1098, "path"=w1099) -> ("file or folder exists?"=w1096:bool, "dup path"=w1097:path)  [unwired: 7 in, 1 out]
            n518 = invoke on="Image Out" class="ImageControl" method="Clear ROI"() -> ()  [unwired: 3 in, 3 out]
            n519 = case shown="True" w1096 {
              tunnel: w1097 -> [_ w1165]
              frame False {
              }
              frame True {
                n520 = Read from Text File(file (use dialog)=w1165) -> (text=w1169:string)  [unwired: 3 in, 3 out]
                n521 = property on="Image Out" class="ImageControl"() -> ("ROI"=w1166:T9)  [unwired: 2 in, 2 out]
                n522 = Unflatten From String(type=w1166, binary string=w1169) -> (value=w1167:T9, error out=w1168:errorcluster)  [unwired: 3 in, 1 out]
                n523 = property on="Image Out" class="ImageControl"(error in=w1168, "ROI"=w1167) -> ()  [unwired: 1 in, 2 out]
              }
            }
          }
          event "Up Button": Mouse Down {
            w1384 = 0
            n524 = event-data() -> ()  [unwired: 1 in, 5 out]
            n525 = local read "Data File"() -> (w1314:path)
            n526 = call "Recorded Values.vi"("Path"=w1314) -> ("Recorded Char"=w1312:T5, "Recorded Prop"=w1311:T6, "Fabrication Prop"=w1313:T7)  [unwired: 8 in]
            n527 = Unbundle By Name(w1312) -> ("Mobility-Sat"=w1298:dbl, "Moblitity-Lin"=w1297:dbl, "On/Off"=w1296:dbl, "Threshold Voltage"=w1295:dbl, "Onset Voltage"=w1294:dbl, "STS"=w1293:dbl, "Trap Density-VT"=w1292:dbl, "Trap Density-STS"=w1291:dbl)
            n528 = Unbundle By Name(w1313) -> ("Date Created"=w1290:string, "Material"=w1310:string, "Solvent"=w1309:string, "Concentration"=w1308:dbl, "Method"=w1307:string, "Dielectric (nm)"=w1306:dbl, "Treatment"=w1305:string, "Comments"=w1304:string)
            n529 = Unbundle By Name(w1311) -> ("Date Recorded"=w1303:string, "Index"=w1302:string, "Length"=w1301:dbl, "Width"=w1300:dbl, "Sample Temp"=w1299:dbl)
            n530 = local read "Data File"() -> (w1380:path)
            n531 = local read "NumPts 2"() -> (w1350:dbl)
            n532 = local write "Date Created"(w1290) -> ()
            n533 = local write "Rec: Material"(w1310) -> ()
            n534 = local write "Rec: Solvent"(w1309) -> ()
            n535 = local write "Rec: Concentration"(w1308) -> ()
            n536 = local write "Rec: Method"(w1307) -> ()
            n537 = local write "Rec: Dielectric (d)"(w1306) -> ()
            n538 = local write "Surface Treatment:"(w1305) -> ()
            n539 = local write "Comments"(w1304) -> ()
            n540 = local write "Index"(w1302) -> ()
            n541 = local write "Rec: Mobility-Sat"(w1298) -> ()
            n542 = local write "Rec: Mobility-Lin"(w1297) -> ()
            n543 = local write "Rec: On/Off"(w1296) -> ()
            n544 = local write "Rec: VT"(w1295) -> ()
            n545 = local write "Rec: Onset V"(w1294) -> ()
            n546 = local write "Rec: STS"(w1293) -> ()
            n547 = local write "Rec: Trap Density-VT"(w1292) -> ()
            n548 = local write "Rec: Trap Density-STS"(w1291) -> ()
            n549 = local read "NumPts"() -> (w1355:dbl)
            n550 = local write "Date Recorded"(w1303) -> ()
            n551 = local write "Rec: Length"(w1301) -> ()
            n552 = local write "Rec: Width"(w1300) -> ()
            n553 = local write "Rec: Temp"(w1299) -> ()
            n554 = local read "Folder Index"() -> (w1316:dbl)
            n555 = property on="Image Out" class="ImageControl"() -> (error out=w1319:errorcluster, "Image Center Position"=w1323:cluster{"X":u32, "Y":u32})  [unwired: 2 in, 1 out]
            n556 = Strip Path(path=w1380) -> (stripped path=w1379:path, name=w1398:string)
            n557 = local write "Data Folder"(w1379) -> ()
            n558 = List Folder(path=w1379) -> (filenames=w1389:string[], error out=w1329:errorcluster)  [unwired: 3 in, 2 out]
            n559 = Path To String(path=w1379) -> (string=w1399:string)
            n560 = Search 1D Array(1D array=w1389, element=w1398) -> (index of element=w1390:i32)  [unwired: 1 in]
            n561 = Unbundle(w1323) -> ("X"=w1321:u32)  [unwired: 1 out]
            n562 = Equal To 0?(x=w1390) -> (x = 0?=w1391:bool)
            n563 = Bundle("X"=w1321, 0) -> (w1322:cluster{"X":u32, i32})  [unwired: 1 in]
            n564 = property on="Image Out" class="ImageControl"(error in=w1319, "Image Center Position"=w1322) -> ()  [unwired: 1 in, 2 out]
            n565 = Array Size(array=w1389) -> (size(s)=w1317:i32)
            n566 = case shown="True" w1391 {
              tunnel: w1316 -> [w1526 _]
              tunnel: [w1525 w1527] -> w1315
              tunnel: w1317 -> [_ w1528]
              frame False {
                n567 = Decrement(x=w1526) -> (x-1=w1525:dbl)
              }
              frame True {
                n568 = Decrement(x=w1528) -> (x-1=w1527:i32)
              }
            }
            n569 = Index Array(array=w1389, index=w1315) -> (element=w1392:string)
            n570 = local write "Data Name:"(w1392) -> ()
            n571 = local write "Folder Index"(w1315) -> ()
            n572 = Concatenate Strings(w1399, "\\", w1392) -> (w1397:string)
            n573 = String To Path(string=w1397) -> (path=w1356:path)
            n574 = call "sub_thresh_swing_subvi.vi"("Path"=w1356, "NumPts"=w1350) -> ("Index"=w1349:dbl, "XY Graph"=w1345:cluster{dbl[], dbl[]}[], "Sub Threshold Swing"=w1357:dbl)  [unwired: 9 in, 2 out]
            n575 = Decimate 1D Array(w1345) -> (w1348:cluster{dbl[], dbl[]}[])  [unwired: 1 out]
            n576 = Array To Cluster(array=w1348) -> (cluster=w1346:T8)
            n577 = Unbundle(w1346) -> ("[0]"=w1347:cluster{dbl[], dbl[]})  [unwired: 8 out]
            n578 = Unbundle(w1347) -> (w1344:dbl[], w1343:dbl[])
            n579 = Array Subset(array=w1344, index=w1349, length=w1350) -> (w1352:dbl[])
            n580 = Array Subset(array=w1343, index=w1349, length=w1350) -> (w1351:dbl[])
            n581 = local write "Calc: STS"(w1357) -> ()
            n582 = local write "Array 8"(w1352) -> ()
            n583 = local write "Array 7"(w1351) -> ()
            n584 = call "mobility_subvi_07_12a_JW.vi"("Path"=w1356, "NumPts"=w1355) -> ("Dielectric (d)"=w1359:dbl, "Index"=w1361:dbl, "XY Graph"=w1367:cluster{dbl[], dbl[]}[], "Length"=w1358:dbl, "Vt"=w1360:dbl, "Width"=w1340:dbl, "Table Control"=w1395:string[][], "Table Control 2"=w1394:string[][], "Mobility"=w1393:dbl)  [unwired: 4 in, 1 out]
            n585 = local write "New: Length"(w1358) -> ()
            n586 = local write "New: Dielectric"(w1359) -> ()
            n587 = local write "New: Width"(w1340) -> ()
            n588 = local write "Table Control"(w1395) -> ()
            n589 = Decimate 1D Array(w1367) -> (w1368:cluster{dbl[], dbl[]}[])  [unwired: 1 out]
            n590 = local write "XY Graph 2"(w1345) -> ()
            n591 = local write "Calc: Mobility-Sat"(w1393) -> ()
            n592 = Array To Cluster(array=w1368) -> (cluster=w1370:T8)
            n593 = local write "XY Graph"(w1367) -> ()
            n594 = local write "Index 2"(w1349) -> ()
            n595 = local write "Table Control 2"(w1394) -> ()
            n596 = Unbundle(w1370) -> ("[0]"=w1369:cluster{dbl[], dbl[]})  [unwired: 8 out]
            n597 = Unbundle(w1369) -> (w1354:dbl[], w1353:dbl[])
            n598 = local write "Calc: VT"(w1360) -> ()
            n599 = Array Subset(array=w1354, index=w1361, length=w1355) -> (w1366:dbl[])
            n600 = Array Subset(array=w1353, index=w1361, length=w1355) -> (w1365:dbl[])
            n601 = local write "Array 2"(w1365) -> ()
            n602 = local write "Array"(w1366) -> ()
            n603 = local write "MobVi Index"(w1361) -> ()
            n604 = local write "Data File"(w1356) -> ()
            n605 = local read "Image Folder"() -> (w1318:path)
            n606 = local write "Slide"(w1361) -> ()
            n607 = List Folder(path=w1318, error in=w1329) -> (filenames=w1378:string[], error out=w1328:errorcluster)  [unwired: 2 in, 2 out]
            n608 = call-poly <vilib>:"Read From Spreadsheet File.vi"("file path (dialog if empty)"=w1356) -> ("all rows"=w1386:string[][])  [unwired: 6 in, 4 out]
            n609 = Array Size(array=w1386) -> (size(s)=w1385:i32[])
            n610 = Index Array(array=w1385, index=w1384) -> (element=w1363:i32)
            n611 = Subtract(x=w1363, y=20) -> (x-y=w1362:i32)
            n612 = property on="Slide" class="Slide (strict)"("Scale.Maximum"=w1362) -> ()  [unwired: 2 in, 2 out]
            n613 = Array Subset(array=w1386, index (row)=w1384, index (col)=w1384, length (col)=3) -> (w1387:string[][])  [unwired: 1 in]
            n614 = Reshape Array(w1387, w1363) -> (w1373:string[])
            n615 = Search 1D Array(1D array=w1373, element="Mobility-Sat (cm^2/Vs):") -> (index of element=w1376:i32)  [unwired: 1 in]
            n616 = Increment(x=w1376) -> (x+1=w1375:i32)
            n617 = Index Array(array=w1373, index=w1375) -> (element=w1372:string)
            n618 = Fract/Exp String To Number(string=w1372) -> (number=w1371:dbl)  [unwired: 3 in, 1 out]
            n619 = local write "Rec: Mobility-Sat"(w1371) -> ()
            n620 = Search 1D Array(1D array=w1373, element="Index:") -> (index of element=w1381:i32)  [unwired: 1 in]
            n621 = Increment(x=w1381) -> (x+1=w1382:i32)
            n622 = Index Array(array=w1373, index=w1382) -> (element=w1325:string)
            n623 = while {
              tunnel: w1378 -> [w1412]
              tunnel: w1325 -> [w1410]
              tunnel: [w1409] -> w1377
              tunnel: w1363 -> [w1408]
              i -> [w1409]
              stop <- w1405 stop-if-true
              n624 = Index Array(array=w1412, index=w1409) -> (element=w1413:string)
              n625 = xnode "Match Regular Expression"("input string"=w1413, "regular expression"=w1410) -> ("whole match"=w1411:string)  [unwired: 4 in, 4 out]
              n626 = Equal?(x=w1411, y=w1410) -> (x = y?=w1407:bool)
              n627 = Equal?(x=w1408, y=w1409) -> (x = y?=w1406:bool)
              n628 = Or(x=w1407, y=w1406) -> (x .or. y?=w1405:bool)
            }
            n629 = local write "Index"(w1325) -> ()
            n630 = Build Path(base path=w1318, name or relative path="ROI") -> (appended path=w1326:path)
            n631 = Build Path(base path=w1326, name or relative path=w1325) -> (appended path=w1324:path)
            n632 = invoke on="Image Out" class="ImageControl" method="Clear ROI"(error in=w1328) -> (error out=w1332:errorcluster)  [unwired: 2 in, 2 out]
            n633 = call <vilib>:"Check if File or Folder Exists.vi"("error in (no error)"=w1332, "path"=w1324) -> ("file or folder exists?"=w1330:bool, "dup path"=w1331:path)  [unwired: 7 in, 1 out]
            n634 = local read "No Image"() -> (w1341:path)
            n635 = Index Array(array=w1378, index=w1377) -> (element=w1334:string)
            n636 = Build Path(base path=w1318, name or relative path=w1334) -> (appended path=w1333:path)
            n637 = local write "Image Name"(w1334) -> ()
            n638 = case shown="True" w1330 {
              tunnel: w1331 -> [_ w1400]
              frame False {
              }
              frame True {
                n639 = Read from Text File(file (use dialog)=w1400) -> (text=w1404:string)  [unwired: 3 in, 3 out]
                n640 = property on="Image Out" class="ImageControl"() -> ("ROI"=w1401:T9)  [unwired: 2 in, 2 out]
                n641 = Unflatten From String(type=w1401, binary string=w1404) -> (value=w1402:T9, error out=w1403:errorcluster)  [unwired: 3 in, 1 out]
                n642 = property on="Image Out" class="ImageControl"(error in=w1403, "ROI"=w1402) -> ()  [unwired: 1 in, 2 out]
              }
            }
            n643 = Empty String/Path?(string/path=w1334) -> (empty?=w1342:bool)
            n644 = Select(t=w1341, s=w1342, f=w1333) -> (s? t:f=w1335:path)
            n645 = call "Vision Acquisition5"("Image Path"=w1335) -> ("Image Out"=w1339:T2)  [unwired: 25 in, 1 out]
            n646 = local write "Image File"(w1335) -> ()
            n647 = local write "Image Out 2"(w1339) -> ()
            n648 = local write "Image Out"(w1339) -> ()
            n649 = call <vilib>:"Get File Extension.vi"("file"=w1335) -> ("lowercase file extension"=w1337:string)  [unwired: 7 in, 3 out]
            n650 = local write "String"(w1337) -> ()
            n651 = Search 1D Array(1D array=string[] ["bmp", "jpeg", "png", "jpg", "gif"], element=w1337) -> (index of element=w1336:i32)  [unwired: 1 in]
            n652 = Less Than 0?(x=w1336) -> ()  [unwired: 1 out]
          }
          event "Save Changes? 3": Mouse Down {
            n653 = event-data() -> ()  [unwired: 1 in, 7 out]
            n654 = local read "Image Folder"() -> (w1529:path)
            n655 = Build Path(base path=w1529, name or relative path="ROI") -> (appended path=w1536:path)
            n656 = call <vilib>:"Check if File or Folder Exists.vi"("path"=w1536) -> ("file or folder exists?"=w1538:bool, "dup path"=w1535:path)  [unwired: 8 in, 1 out]
            n657 = case shown="False" w1538 {
              tunnel: w1535 -> [w1540 w1541]
              tunnel: [w1539 w1541] -> w1530
              frame False {
                n658 = Create Folder(path (use dialog)=w1540) -> (created path=w1539:path)  [unwired: 2 in, 2 out]
              }
              frame True {
              }
            }
            n659 = property on="Image Out" class="ImageControl"() -> ("ROI"=w1534:T9)  [unwired: 2 in, 2 out]
            n660 = local read "Index"() -> (w1532:string)
            n661 = Flatten To String(anything=w1534) -> (data string=w1533:string)  [unwired: 3 in, 2 out]
            n662 = Build Path(base path=w1530, name or relative path=w1532) -> (appended path=w1531:path)
            n663 = Write to Text File(file (use dialog)=w1531, text=w1533) -> ()  [unwired: 2 in, 3 out]
          }
          event "Next Button": Mouse Down {
            n664 = event-data() -> ()  [unwired: 1 in, 5 out]
            n665 = local read "XY Graph"() -> (w1554:cluster{dbl[], dbl[]}[])
            n666 = local read "MobVi Index"() -> (w1556:dbl)
            n667 = local read "NumPts"() -> (w1555:dbl)
            n668 = Decimate 1D Array(w1554) -> (w1550:cluster{dbl[], dbl[]}[], w1549:cluster{dbl[], dbl[]}[])
            n669 = Array To Cluster(array=w1550) -> (cluster=w1560:T8)
            n670 = Unbundle(w1560) -> ("[0]"=w1559:cluster{dbl[], dbl[]})  [unwired: 8 out]
            n671 = Increment(x=w1556) -> (x+1=w1551:dbl)
            n672 = Unbundle(w1559) -> (w1558:dbl[], w1557:dbl[])
            n673 = local write "MobVi Index"(w1551) -> ()
            n674 = Array Subset(array=w1558, index=w1551, length=w1555) -> (w1547:dbl[])
            n675 = Array Subset(array=w1557, index=w1551, length=w1555) -> (w1546:dbl[])
            n676 = Bundle(w1547, w1546) -> (w1553:cluster{dbl[], dbl[]})  [unwired: 1 in]
            n677 = Build Array (concatenate)(w1550, w1549, w1553) -> (w1552:cluster{dbl[], dbl[]}[])
            n678 = local write "XY Graph"(w1552) -> ()
            n679 = local read "New: Dielectric"() -> (w1545:dbl)
            n680 = local write "Array 2"(w1546) -> ()
            n681 = local read "New: Length"() -> (w1544:dbl)
            n682 = local write "Array"(w1547) -> ()
            n683 = local read "New: Width"() -> (w1543:dbl)
            n684 = call "mob_calc_subvi.vi"("Width"=w1543, "Length"=w1544, "Dielectric (d)"=w1545, "Array 2"=w1546, "Array"=w1547) -> ("Vt"=w1542:dbl, "Mobility"=w1548:dbl)  [unwired: 4 in, 1 out]
            n685 = local write "New: Mobility-Sat"(w1548) -> ()
            n686 = local write "New: VT"(w1542) -> ()
          }
          event "Next Button 2": Mouse Down {
            n687 = event-data() -> ()  [unwired: 1 in, 7 out]
            n688 = local read "XY Graph 2"() -> (w1569:cluster{dbl[], dbl[]}[])
            n689 = local read "Index 2"() -> (w1571:dbl)
            n690 = local read "NumPts 2"() -> (w1570:dbl)
            n691 = Decimate 1D Array(w1569) -> (w1565:cluster{dbl[], dbl[]}[], w1564:cluster{dbl[], dbl[]}[])
            n692 = Array To Cluster(array=w1565) -> (cluster=w1575:T8)
            n693 = Unbundle(w1575) -> ("[0]"=w1574:cluster{dbl[], dbl[]})  [unwired: 8 out]
            n694 = Increment(x=w1571) -> (x+1=w1566:dbl)
            n695 = Unbundle(w1574) -> (w1573:dbl[], w1572:dbl[])
            n696 = local write "Index 2"(w1566) -> ()
            n697 = Array Subset(array=w1573, index=w1566, length=w1570) -> (w1562:dbl[])
            n698 = Array Subset(array=w1572, index=w1566, length=w1570) -> (w1561:dbl[])
            n699 = Bundle(w1562, w1561) -> (w1568:cluster{dbl[], dbl[]})  [unwired: 1 in]
            n700 = Build Array (concatenate)(w1565, w1564, w1568) -> (w1567:cluster{dbl[], dbl[]}[])
            n701 = local write "XY Graph 2"(w1567) -> ()
            n702 = local write "Array 8"(w1562) -> ()
            n703 = call "sts_calc_subvi.vi"("Array 2"=w1562, "Array"=w1561) -> ("STS"=w1563:dbl)  [unwired: 9 in]
            n704 = local write "Array 7"(w1561) -> ()
            n705 = local write "New: STS"(w1563) -> ()
          }
          event "Previous Button 2": Mouse Down {
            n706 = event-data() -> ()  [unwired: 1 in, 7 out]
            n707 = local read "XY Graph 2"() -> (w1585:cluster{dbl[], dbl[]}[])
            n708 = local read "NumPts 2"() -> (w1586:dbl)
            n709 = local read "Index 2"() -> (w1578:dbl)
            n710 = Decimate 1D Array(w1585) -> (w1582:cluster{dbl[], dbl[]}[], w1581:cluster{dbl[], dbl[]}[])
            n711 = Array To Cluster(array=w1582) -> (cluster=w1590:T8)
            n712 = Unbundle(w1590) -> ("[0]"=w1589:cluster{dbl[], dbl[]})  [unwired: 8 out]
            n713 = Decrement(x=w1578) -> (x-1=w1579:dbl)
            n714 = Unbundle(w1589) -> (w1588:dbl[], w1587:dbl[])
            n715 = local write "Index 2"(w1579) -> ()
            n716 = Array Subset(array=w1588, index=w1579, length=w1586) -> (w1576:dbl[])
            n717 = Array Subset(array=w1587, index=w1579, length=w1586) -> (w1577:dbl[])
            n718 = Bundle(w1576, w1577) -> (w1584:cluster{dbl[], dbl[]})  [unwired: 1 in]
            n719 = Build Array (concatenate)(w1582, w1581, w1584) -> (w1583:cluster{dbl[], dbl[]}[])
            n720 = local write "XY Graph 2"(w1583) -> ()
            n721 = local write "Array 7"(w1577) -> ()
            n722 = call "sts_calc_subvi.vi"("Array 2"=w1576, "Array"=w1577) -> ("STS"=w1580:dbl)  [unwired: 9 in]
            n723 = local write "Array 8"(w1576) -> ()
            n724 = local write "New: STS"(w1580) -> ()
          }
          event "Previous Button": Mouse Down {
            n725 = event-data() -> ()  [unwired: 1 in, 5 out]
            n726 = local read "XY Graph"() -> (w1604:cluster{dbl[], dbl[]}[])
            n727 = Decimate 1D Array(w1604) -> (w1601:cluster{dbl[], dbl[]}[], w1600:cluster{dbl[], dbl[]}[])
            n728 = local read "MobVi Index"() -> (w1599:dbl)
            n729 = local read "NumPts"() -> (w1605:dbl)
            n730 = Array To Cluster(array=w1601) -> (cluster=w1609:T8)
            n731 = Unbundle(w1609) -> ("[0]"=w1608:cluster{dbl[], dbl[]})  [unwired: 8 out]
            n732 = Decrement(x=w1599) -> (x-1=w1598:dbl)
            n733 = Unbundle(w1608) -> (w1607:dbl[], w1606:dbl[])
            n734 = local read "New: Dielectric"() -> (w1592:dbl)
            n735 = Array Subset(array=w1607, index=w1598, length=w1605) -> (w1597:dbl[])
            n736 = local write "MobVi Index"(w1598) -> ()
            n737 = Array Subset(array=w1606, index=w1598, length=w1605) -> (w1596:dbl[])
            n738 = Bundle(w1597, w1596) -> (w1603:cluster{dbl[], dbl[]})  [unwired: 1 in]
            n739 = Build Array (concatenate)(w1601, w1600, w1603) -> (w1602:cluster{dbl[], dbl[]}[])
            n740 = local write "XY Graph"(w1602) -> ()
            n741 = local read "New: Length"() -> (w1593:dbl)
            n742 = local write "Array 2"(w1596) -> ()
            n743 = local read "New: Width"() -> (w1594:dbl)
            n744 = call "mob_calc_subvi.vi"("Width"=w1594, "Length"=w1593, "Dielectric (d)"=w1592, "Array 2"=w1596, "Array"=w1597) -> ("Vt"=w1591:dbl, "Mobility"=w1595:dbl)  [unwired: 4 in, 1 out]
            n745 = local write "New: Mobility-Sat"(w1595) -> ()
            n746 = local write "Array"(w1597) -> ()
            n747 = local write "New: VT"(w1591) -> ()
          }
          event "Slide": Value Change {
            n748 = event-data() -> ()  [unwired: 1 in, 5 out]
            n749 = local read "XY Graph"() -> (w1622:cluster{dbl[], dbl[]}[])
            n750 = local read "Slide"() -> (w1611:dbl)
            n751 = Decimate 1D Array(w1622) -> (w1619:cluster{dbl[], dbl[]}[], w1618:cluster{dbl[], dbl[]}[])
            n752 = local read "NumPts"() -> (w1623:dbl)
            n753 = Array To Cluster(array=w1619) -> (cluster=w1627:T8)
            n754 = Unbundle(w1627) -> ("[0]"=w1626:cluster{dbl[], dbl[]})  [unwired: 8 out]
            n755 = Unbundle(w1626) -> (w1625:dbl[], w1624:dbl[])
            n756 = local read "New: Dielectric"() -> (w1612:dbl)
            n757 = Array Subset(array=w1625, index=w1611, length=w1623) -> (w1617:dbl[])
            n758 = local write "MobVi Index"(w1611) -> ()
            n759 = Array Subset(array=w1624, index=w1611, length=w1623) -> (w1616:dbl[])
            n760 = Bundle(w1617, w1616) -> (w1621:cluster{dbl[], dbl[]})  [unwired: 1 in]
            n761 = Build Array (concatenate)(w1619, w1618, w1621) -> (w1620:cluster{dbl[], dbl[]}[])
            n762 = local write "XY Graph"(w1620) -> ()
            n763 = local read "New: Length"() -> (w1613:dbl)
            n764 = local write "Array 2"(w1616) -> ()
            n765 = local read "New: Width"() -> (w1614:dbl)
            n766 = call "mob_calc_subvi.vi"("Width"=w1614, "Length"=w1613, "Dielectric (d)"=w1612, "Array 2"=w1616, "Array"=w1617) -> ("Vt"=w1610:dbl, "Mobility"=w1615:dbl)  [unwired: 4 in, 1 out]
            n767 = local write "New: Mobility-Sat"(w1615) -> ()
            n768 = local write "Array"(w1617) -> ()
            n769 = local write "New: VT"(w1610) -> ()
          }
          event "Slide 2": Value Change {
            n770 = event-data() -> ()  [unwired: 1 in, 5 out]
            n771 = local read "XY Graph 2"() -> (w1636:cluster{dbl[], dbl[]}[])
            n772 = local read "Slide 2"() -> (w1631:dbl)
            n773 = Decimate 1D Array(w1636) -> (w1633:cluster{dbl[], dbl[]}[], w1632:cluster{dbl[], dbl[]}[])
            n774 = local read "NumPts 2"() -> (w1637:dbl)
            n775 = Array To Cluster(array=w1633) -> (cluster=w1641:T8)
            n776 = Unbundle(w1641) -> ("[0]"=w1640:cluster{dbl[], dbl[]})  [unwired: 8 out]
            n777 = Unbundle(w1640) -> (w1639:dbl[], w1638:dbl[])
            n778 = Array Subset(array=w1639, index=w1631, length=w1637) -> (w1629:dbl[])
            n779 = Array Subset(array=w1638, index=w1631, length=w1637) -> (w1628:dbl[])
            n780 = local write "Index 2"(w1631) -> ()
            n781 = Bundle(w1629, w1628) -> (w1635:cluster{dbl[], dbl[]})  [unwired: 1 in]
            n782 = Build Array (concatenate)(w1633, w1632, w1635) -> (w1634:cluster{dbl[], dbl[]}[])
            n783 = local write "XY Graph 2"(w1634) -> ()
            n784 = local write "Array 7"(w1628) -> ()
            n785 = local write "Array 8"(w1629) -> ()
            n786 = call "sts_calc_subvi.vi"("Array 2"=w1629, "Array"=w1628) -> ("STS"=w1630:dbl)  [unwired: 9 in]
            n787 = local write "New: STS"(w1630) -> ()
          }
          event "Save Changes?": Mouse Down {
            n788 = event-data() -> ()  [unwired: 1 in, 5 out]
            n789 = flat-sequence {
              tunnel: [w1672] -> w1647
              tunnel: [w1671] -> w1645
              tunnel: [w1671] -> w1644
              tunnel: [w1654] -> w1642
              tunnel: w1647 -> [w1785]
              tunnel: [w1786] -> w1646
              tunnel: w1645 -> [w1786]
              tunnel: w1644 -> [w1784]
              tunnel: [w1782] -> w1643
              tunnel: w1642 -> [w1782]
              tunnel: w1646 -> [w1791]
              tunnel: w1643 -> [w1790]
              frame #0 {
                w1659 = -1
                w1652 = "S.T.S. (V/decade):"
                w1653 = "Threshold V (V):"
                (unwired) 3
                w1657 = 1
                n790 = local read "New: Mobility-Sat"() -> (w1694:dbl)
                n791 = local read "Data File"() -> (w1672:path)
                n792 = local read "New: Width"() -> (w1685:dbl)
                n793 = local read "New: Dielectric"() -> (w1695:dbl)
                n794 = local read "New: Length"() -> (w1683:dbl)
                n795 = flat-sequence {
                  tunnel: [w1713] -> w1651
                  tunnel: w1651 -> [w1730]
                  frame #0 {
                    # "Makes Empty File for Transformer Data"
                    n796 = local read "Data Folder"() -> (w1702:path)
                    n797 = Build Path(base path=w1702, name or relative path="Stats") -> (appended path=w1704:path)
                    n798 = call <vilib>:"Check if File or Folder Exists.vi"("path"=w1704) -> ("file or folder exists?"=w1705:bool, "dup path"=w1706:path)  [unwired: 8 in, 1 out]
                    n799 = case shown="False" w1705 {
                      tunnel: [w1710 w1712] -> w1707
                      tunnel: w1706 -> [w1711 w1712]
                      frame False {
                        n800 = Create Folder(path (use dialog)=w1711) -> (created path=w1710:path)  [unwired: 2 in, 2 out]
                      }
                      frame True {
                      }
                    }
                    n801 = Build Path(base path=w1707, name or relative path="Tranformer Data.txt") -> (appended path=w1709:path)
                    n802 = call-poly <vilib>:"Write To Spreadsheet File.vi"("append to file? (new file:F)"=TRUE, "file path (dialog if empty)"=w1709) -> ()  [unwired: 6 in, 1 out]
                  }
                  frame #1 {
                    # "Adds Headers if they don't exist"
                    n803 = Concatenate Strings("Stats\\", "Tranformer Data.txt") -> (w1720:string)
                    n804 = local read "Data Folder"() -> (w1719:path)
                    n805 = Build Path(base path=w1719, name or relative path=w1720) -> (appended path=w1713:path)
                    n806 = call-poly <vilib>:"Read From Spreadsheet File.vi"("file path (dialog if empty)"=w1713) -> ("first row"=w1718:string[])  [unwired: 6 in, 4 out]
                    n807 = Search 1D Array(1D array=w1718, element="DeviceID") -> (index of element=w1716:i32)  [unwired: 1 in]
                    n808 = Equal?(x=w1716, y=0) -> (x = y?=w1714:bool)
                    n809 = case shown="False" w1714 {
                      tunnel: w1713 -> [w1724 _]
                      frame False {
                        n810 = local read "Transformer \nHeaders"() -> (w1723:string[])
                        n811 = call-poly <vilib>:"Write To Spreadsheet File.vi"("1D data"=w1723, "file path (dialog if empty)"=w1724) -> ()  [unwired: 6 in, 1 out]
                      }
                      frame True {
                      }
                    }
                  }
                  frame #2 {
                    # "Adds current device if it doesn't exist"
                    n812 = local read "Current \nRecord"() -> (w1729:string[])
                    n813 = Index Array(array=w1729, index=0) -> (element=w1728:string)
                    n814 = Concatenate Strings("Stats\\", "Tranformer Data.txt") -> (w1733:string)
                    n815 = local read "Data Folder"() -> (w1732:path)
                    n816 = local write "Current Device ID"(w1728) -> ()
                    n817 = local read "Current Device ID"() -> (w1738:string)
                    n818 = Build Path(base path=w1732, name or relative path=w1733) -> (appended path=w1731:path)
                    n819 = call-poly <vilib>:"Read From Spreadsheet File.vi"("file path (dialog if empty)"=w1731) -> ("all rows"=w1725:string[][])  [unwired: 6 in, 4 out]
                    n820 = Index Array(array=w1725, index (col)=0) -> (element=w1726:string[])  [unwired: 1 in]
                    n821 = Search 1D Array(1D array=w1726, element=w1738) -> (index of element=w1727:i32)  [unwired: 1 in]
                    n822 = Equal?(x=w1727, y=-1) -> (x = y?=w1740:bool)
                    n823 = case shown="False" w1740 {
                      tunnel: w1730 -> [w1743 w1754]
                      tunnel: w1727 -> [w1746 _]
                      tunnel: w1725 -> [w1747 _]
                      frame False {
                        n824 = local read "Current \nRecord"() -> (w1745:string[])
                        n825 = Replace Array Subset(array=w1747, new element=w1745, index (row)=w1746) -> (w1744:string[][])  [unwired: 1 in]
                        n826 = flat-sequence {
                          tunnel: w1743 -> [w1748]
                          tunnel: w1744 -> [w1749]
                          tunnel: [w1749] -> w1742
                          tunnel: [w1748] -> w1741
                          tunnel: w1742 -> [w1751]
                          tunnel: w1741 -> [w1750]
                          frame #0 {
                            n827 = Delete(path (use dialog)=w1748) -> ()  [unwired: 4 in, 3 out]
                          }
                          frame #1 {
                            n828 = call-poly <vilib>:"Write To Spreadsheet File.vi"("append to file? (new file:F)"=TRUE, "2D data"=w1751, "file path (dialog if empty)"=w1750) -> ()  [unwired: 5 in, 1 out]
                          }
                        }
                      }
                      frame True {
                        n829 = local read "Current \nRecord"() -> (w1753:string[])
                        n830 = call-poly <vilib>:"Write To Spreadsheet File.vi"("append to file? (new file:F)"=TRUE, "1D data"=w1753, "file path (dialog if empty)"=w1754) -> ()  [unwired: 5 in, 1 out]
                      }
                    }
                  }
                }
                n831 = call-poly <vilib>:"Read From Spreadsheet File.vi"("file path (dialog if empty)"=w1672) -> ("all rows"=w1664:string[][])  [unwired: 6 in, 4 out]
                n832 = Number To Fractional String(number=w1683) -> (F-format string=w1675:string)  [unwired: 3 in]
                n833 = Replace Array Subset(array=w1664, new element=w1675, index (row)=12, index (col)=w1657) -> (w1679:string[][])
                n834 = Number To Fractional String(number=w1685) -> (F-format string=w1686:string)  [unwired: 3 in]
                n835 = Replace Array Subset(array=w1679, new element=w1686, index (row)=13, index (col)=w1657) -> (w1681:string[][])
                n836 = Number To Fractional String(number=w1694) -> (F-format string=w1673:string)  [unwired: 3 in]
                n837 = Number To Fractional String(number=w1695) -> (F-format string=w1674:string)  [unwired: 3 in]
                n838 = Number To Decimal String(number=w1683) -> (decimal integer string=w1682:string)  [unwired: 1 in]
                n839 = local read "Rec: Temp"() -> (w1650:dbl)
                n840 = Equal To 0?(x=w1650) -> (x = 0?=w1649:bool)
                n841 = case shown="False" w1649 {
                  tunnel: [w1696 ""] -> w1648
                  frame False {
                    n842 = local read "Rec: Temp"() -> (w1699:dbl)
                    n843 = Number To Decimal String(number=w1699) -> (decimal integer string=w1698:string)  [unwired: 1 in]
                    n844 = Concatenate Strings(w1698, "K") -> (w1696:string)
                  }
                  frame True {
                  }
                }
                n845 = Strip Path(path=w1672) -> (stripped path=w1693:path)  [unwired: 1 out]
                n846 = local read "Index"() -> (w1688:string)
                n847 = Replace Array Subset(array=w1681, new element=w1673, index (row)=15, index (col)=w1657) -> (w1680:string[][])
                n848 = Number To Decimal String(number=w1685) -> (decimal integer string=w1684:string)  [unwired: 1 in]
                n849 = Path To String(path=w1693) -> (string=w1691:string)
                n850 = Replace Array Subset(array=w1680, new element=w1674, index (row)=7, index (col)=w1657) -> (w1656:string[][])
                n851 = call "Build Text"("Temp"=w1648, "Index"=w1688, "Length"=w1682, "Width"=w1684) -> ("Result"=w1689:string)  [unwired: 10 in, 1 out]
                n852 = Concatenate Strings(w1691, "\\", w1689) -> (w1690:string)
                n853 = String To Path(string=w1690) -> (path=w1671:path)
                n854 = Array Size(array=w1664) -> (size(s)=w1666:i32[])
                n855 = Index Array(array=w1666, index=0) -> (element=w1665:i32)
                n856 = Array Subset(array=w1664, index (row)=0, index (col)=0) -> (w1670:string[][])  [unwired: 2 in]
                n857 = Reshape Array(w1670, w1665) -> (w1658:string[])
                n858 = Search 1D Array(1D array=w1658, element=w1653) -> (index of element=w1662:i32)  [unwired: 1 in]
                n859 = Search 1D Array(1D array=w1658, element=w1652) -> (index of element=w1663:i32)  [unwired: 1 in]
                n860 = Equal?(x=w1662, y=w1659) -> (x = y?=w1660:bool)
                n861 = Equal?(x=w1663, y=w1659) -> (x = y?=w1661:bool)
                n862 = case shown="True" w1660 {
                  tunnel: w1662 -> [_ _]
                  tunnel: w1656 -> [w1772 w1780]
                  tunnel: [w1771 w1779] -> w1655
                  tunnel: w1653 -> [_ w1778]
                  frame False {
                    n863 = local read "New: VT"() -> (w1774:dbl)
                    n864 = Number To Fractional String(number=w1774) -> (F-format string=w1770:string)  [unwired: 3 in]
                    n865 = Replace Array Subset(array=w1772, new element=w1770, index (row)=17, index (col)=1) -> (w1771:string[][])
                  }
                  frame True {
                    n866 = local read "New: VT"() -> (w1781:dbl)
                    n867 = Number To Fractional String(number=w1781) -> (F-format string=w1777:string)  [unwired: 3 in]
                    n868 = Build Array(w1778, w1777) -> (w1776:string[])
                    n869 = Insert Into Array(array=w1780, index (row)=17, new element=w1776) -> (w1779:string[][])  [unwired: 1 in]
                  }
                }
                n870 = case shown="True" w1661 {
                  tunnel: w1663 -> [_ _]
                  tunnel: w1655 -> [w1759 w1767]
                  tunnel: [w1758 w1766] -> w1654
                  tunnel: w1652 -> [_ w1764]
                  frame False {
                    n871 = local read "New: STS"() -> (w1761:dbl)
                    n872 = Number To Fractional String(number=w1761) -> (F-format string=w1757:string)  [unwired: 3 in]
                    n873 = Replace Array Subset(array=w1759, new element=w1757, index (row)=18, index (col)=1) -> (w1758:string[][])
                  }
                  frame True {
                    n874 = local read "New: STS"() -> (w1768:dbl)
                    n875 = Number To Fractional String(number=w1768) -> (F-format string=w1765:string)  [unwired: 3 in]
                    n876 = Build Array(w1764, w1765) -> (w1763:string[])
                    n877 = Insert Into Array(array=w1767, index (row)=18, new element=w1763) -> (w1766:string[][])  [unwired: 1 in]
                  }
                }
              }
              frame #1 {
                n878 = Equal?(x=w1785, y=w1784) -> (x = y?=w1783:bool)
                n879 = case shown="False" w1783 {
                  tunnel: w1785 -> [w1789 _]
                  tunnel: w1784 -> [w1788 _]
                  frame False {
                    n880 = Move(source path=w1789, 9:TRUE, 10:w1788) -> ()  [unwired: 2 in, 3 out]
                  }
                  frame True {
                  }
                }
              }
              frame #2 {
                n881 = local write "Data File"(w1791) -> ()
                n882 = call-poly <vilib>:"Write To Spreadsheet File.vi"("2D data"=w1790, "file path (dialog if empty)"=w1791) -> ()  [unwired: 6 in, 1 out]
              }
            }
          }
          event "Save Changes? 2": Mouse Down {
            n883 = event-data() -> ()  [unwired: 1 in, 5 out]
            n884 = local read "Data File"() -> (w1816:path)
            n885 = call "Recorded Values.vi"("Path"=w1816) -> ("Recorded Char"=w1814:T5, "Recorded Prop"=w1813:T6, "Fabrication Prop"=w1815:T7)  [unwired: 8 in]
            n886 = Unbundle By Name(w1814) -> ("Mobility-Sat"=w1800:dbl, "Moblitity-Lin"=w1799:dbl, "On/Off"=w1798:dbl, "Threshold Voltage"=w1797:dbl, "Onset Voltage"=w1796:dbl, "STS"=w1795:dbl, "Trap Density-VT"=w1794:dbl, "Trap Density-STS"=w1793:dbl)
            n887 = Unbundle By Name(w1815) -> ("Date Created"=w1792:string, "Material"=w1812:string, "Solvent"=w1811:string, "Concentration"=w1810:dbl, "Method"=w1809:string, "Dielectric (nm)"=w1808:dbl, "Treatment"=w1807:string, "Comments"=w1806:string)
            n888 = Unbundle By Name(w1813) -> ("Date Recorded"=w1805:string, "Index"=w1804:string, "Length"=w1803:dbl, "Width"=w1802:dbl, "Sample Temp"=w1801:dbl)
            n889 = local write "Rec: Material"(w1812) -> ()
            n890 = local write "Date Created"(w1792) -> ()
            n891 = local write "Rec: Solvent"(w1811) -> ()
            n892 = local write "Rec: Concentration"(w1810) -> ()
            n893 = local write "Rec: Method"(w1809) -> ()
            n894 = local write "Rec: Dielectric (d)"(w1808) -> ()
            n895 = local write "Surface Treatment:"(w1807) -> ()
            n896 = local write "Comments"(w1806) -> ()
            n897 = local write "Index"(w1804) -> ()
            n898 = local write "Rec: Mobility-Sat"(w1800) -> ()
            n899 = local write "Rec: Mobility-Lin"(w1799) -> ()
            n900 = local write "Rec: On/Off"(w1798) -> ()
            n901 = local write "Rec: VT"(w1797) -> ()
            n902 = local write "Rec: Onset V"(w1796) -> ()
            n903 = local write "Rec: STS"(w1795) -> ()
            n904 = local write "Rec: Trap Density-VT"(w1794) -> ()
            n905 = local write "Rec: Trap Density-STS"(w1793) -> ()
            n906 = stacked-sequence {
              seq-local: [w1896 _ _ _ _] -> [_ w1954 _ _ _]
              seq-local: [w1895 _ _ _ _] -> [_ w1955 _ _ _]
              seq-local: [w1895 _ _ _ _] -> [_ w1953 _ _ _]
              seq-local: [w1878 _ _ _ _] -> [_ w1951 _ _ _]
              seq-local: [_ w1955 _ _ _] -> [_ _ w1960 _ _]
              seq-local: [_ w1951 _ _ _] -> [_ _ w1959 _ _]
              frame #0 {
                w1883 = -1
                w1876 = "STS (V/decade):"
                w1877 = "Threshold V (V):"
                (unwired) 3
                w1881 = 1
                n907 = local read "Data File"() -> (w1896:path)
                n908 = local read "New: Width"() -> (w1909:dbl)
                n909 = local read "New: Dielectric"() -> (w1919:dbl)
                n910 = local read "New: Length"() -> (w1907:dbl)
                n911 = local read "New: Mobility-Sat"() -> (w1918:dbl)
                n912 = local read "Rec: Temp"() -> (w1875:dbl)
                n913 = call-poly <vilib>:"Read From Spreadsheet File.vi"("file path (dialog if empty)"=w1896) -> ("all rows"=w1888:string[][])  [unwired: 6 in, 4 out]
                n914 = Number To Fractional String(number=w1907) -> (F-format string=w1899:string)  [unwired: 3 in]
                n915 = Replace Array Subset(array=w1888, new element=w1899, index (row)=12, index (col)=w1881) -> (w1903:string[][])
                n916 = Number To Fractional String(number=w1918) -> (F-format string=w1897:string)  [unwired: 3 in]
                n917 = Equal To 0?(x=w1875) -> (x = 0?=w1874:bool)
                n918 = Number To Fractional String(number=w1919) -> (F-format string=w1898:string)  [unwired: 3 in]
                n919 = Number To Fractional String(number=w1909) -> (F-format string=w1910:string)  [unwired: 3 in]
                n920 = Replace Array Subset(array=w1903, new element=w1910, index (row)=13, index (col)=w1881) -> (w1905:string[][])
                n921 = Number To Decimal String(number=w1907) -> (decimal integer string=w1906:string)  [unwired: 1 in]
                n922 = case shown="False" w1874 {
                  tunnel: [w1920 ""] -> w1873
                  frame False {
                    n923 = local read "Rec: Temp"() -> (w1923:dbl)
                    n924 = Number To Decimal String(number=w1923) -> (decimal integer string=w1922:string)  [unwired: 1 in]
                    n925 = Concatenate Strings(w1922, "K") -> (w1920:string)
                  }
                  frame True {
                  }
                }
                n926 = Strip Path(path=w1896) -> (stripped path=w1917:path)  [unwired: 1 out]
                n927 = local read "Index"() -> (w1912:string)
                n928 = Replace Array Subset(array=w1905, new element=w1897, index (row)=15, index (col)=w1881) -> (w1904:string[][])
                n929 = Number To Decimal String(number=w1909) -> (decimal integer string=w1908:string)  [unwired: 1 in]
                n930 = Path To String(path=w1917) -> (string=w1915:string)
                n931 = Replace Array Subset(array=w1904, new element=w1898, index (row)=7, index (col)=w1881) -> (w1880:string[][])
                n932 = call "Build Text2"("Temp"=w1873, "Index"=w1912, "Length"=w1906, "Width"=w1908) -> ("Result"=w1913:string)  [unwired: 10 in, 1 out]
                n933 = Concatenate Strings(w1915, "\\", w1913) -> (w1914:string)
                n934 = String To Path(string=w1914) -> (path=w1895:path)
                n935 = Array Size(array=w1888) -> (size(s)=w1890:i32[])
                n936 = Index Array(array=w1890, index=0) -> (element=w1889:i32)
                n937 = Array Subset(array=w1888, index (row)=0, index (col)=0) -> (w1894:string[][])  [unwired: 2 in]
                n938 = Reshape Array(w1894, w1889) -> (w1882:string[])
                n939 = Search 1D Array(1D array=w1882, element=w1877) -> (index of element=w1886:i32)  [unwired: 1 in]
                n940 = Search 1D Array(1D array=w1882, element=w1876) -> (index of element=w1887:i32)  [unwired: 1 in]
                n941 = Equal?(x=w1886, y=w1883) -> (x = y?=w1884:bool)
                n942 = Equal?(x=w1887, y=w1883) -> (x = y?=w1885:bool)
                n943 = case shown="True" w1884 {
                  tunnel: w1886 -> [_ _]
                  tunnel: w1880 -> [w1941 w1949]
                  tunnel: [w1940 w1948] -> w1879
                  tunnel: w1877 -> [_ w1947]
                  frame False {
                    n944 = local read "New: VT"() -> (w1943:dbl)
                    n945 = Number To Fractional String(number=w1943) -> (F-format string=w1939:string)  [unwired: 3 in]
                    n946 = Replace Array Subset(array=w1941, new element=w1939, index (row)=17, index (col)=1) -> (w1940:string[][])
                  }
                  frame True {
                    n947 = local read "New: VT"() -> (w1950:dbl)
                    n948 = Number To Fractional String(number=w1950) -> (F-format string=w1946:string)  [unwired: 3 in]
                    n949 = Build Array(w1947, w1946) -> (w1945:string[])
                    n950 = Insert Into Array(array=w1949, index (row)=17, new element=w1945) -> (w1948:string[][])  [unwired: 1 in]
                  }
                }
                n951 = case shown="True" w1885 {
                  tunnel: w1887 -> [_ _]
                  tunnel: w1879 -> [w1928 w1936]
                  tunnel: [w1927 w1935] -> w1878
                  tunnel: w1876 -> [_ w1933]
                  frame False {
                    n952 = local read "New: STS"() -> (w1930:dbl)
                    n953 = Number To Fractional String(number=w1930) -> (F-format string=w1926:string)  [unwired: 3 in]
                    n954 = Replace Array Subset(array=w1928, new element=w1926, index (row)=18, index (col)=1) -> (w1927:string[][])
                  }
                  frame True {
                    n955 = local read "New: STS"() -> (w1937:dbl)
                    n956 = Number To Fractional String(number=w1937) -> (F-format string=w1934:string)  [unwired: 3 in]
                    n957 = Build Array(w1933, w1934) -> (w1932:string[])
                    n958 = Insert Into Array(array=w1936, index (row)=18, new element=w1932) -> (w1935:string[][])  [unwired: 1 in]
                  }
                }
              }
              frame #1 {
                n959 = Equal?(x=w1954, y=w1953) -> (x = y?=w1952:bool)
                n960 = case shown="False" w1952 {
                  tunnel: w1954 -> [w1958 _]
                  tunnel: w1953 -> [w1957 _]
                  frame False {
                    n961 = Move(source path=w1958, 9:TRUE, 10:w1957) -> ()  [unwired: 2 in, 3 out]
                  }
                  frame True {
                  }
                }
              }
              frame #2 {
                n962 = local write "Data File"(w1960) -> ()
                n963 = call-poly <vilib>:"Write To Spreadsheet File.vi"("2D data"=w1959, "file path (dialog if empty)"=w1960) -> ()  [unwired: 6 in, 1 out]
              }
              frame #3 {
                w2021 = 0
                # "Moves to next file and displays new image/data"
                n964 = local read "NumPts 2"() -> (w1981:dbl)
                n965 = local read "Folder Index"() -> (w1962:dbl)
                n966 = local read "NumPts"() -> (w1987:dbl)
                n967 = local read "Data File"() -> (w2026:path)
                n968 = property on="Image Out" class="ImageControl"() -> (error out=w1966:errorcluster, "Image Center Position"=w1970:cluster{"X":u32, "Y":u32})  [unwired: 2 in, 1 out]
                n969 = Strip Path(path=w2026) -> (stripped path=w2017:path, name=w2038:string)
                n970 = local write "Data Folder"(w2017) -> ()
                n971 = List Folder(path=w2017) -> (filenames=w2031:string[])  [unwired: 3 in, 3 out]
                n972 = Unbundle(w1970) -> ("X"=w1968:u32)  [unwired: 1 out]
                n973 = Array Size(array=w2031) -> (size(s)=w2027:i32)
                n974 = Path To String(path=w2017) -> (string=w2039:string)
                n975 = Search 1D Array(1D array=w2031, element=w2038) -> (index of element=w2028:i32)  [unwired: 1 in]
                n976 = Bundle("X"=w1968, 0) -> (w1969:cluster{"X":u32, i32})  [unwired: 1 in]
                n977 = Decrement(x=w2027) -> (x-1=w2029:i32)
                n978 = Equal?(x=w2028, y=w2029) -> (x = y?=w2030:bool)
                n979 = case shown="False" w2030 {
                  tunnel: w1962 -> [w2161 _]
                  tunnel: [w2160 0] -> w1961
                  frame False {
                    n980 = Increment(x=w2161) -> (x+1=w2160:dbl)
                  }
                  frame True {
                  }
                }
                n981 = Index Array(array=w2031, index=w1961) -> (element=w2032:string)
                n982 = local write "Data Name:"(w2032) -> ()
                n983 = Concatenate Strings(w2039, "\\", w2032) -> (w2037:string)
                n984 = property on="Image Out" class="ImageControl"(error in=w1966, "Image Center Position"=w1969) -> ()  [unwired: 1 in, 2 out]
                n985 = String To Path(string=w2037) -> (path=w1988:path)
                n986 = call "sub_thresh_swing_subvi.vi"("Path"=w1988, "NumPts"=w1981) -> ("Index"=w1982:dbl, "XY Graph"=w1977:cluster{dbl[], dbl[]}[], "Sub Threshold Swing"=w1989:dbl)  [unwired: 9 in, 2 out]
                n987 = Decimate 1D Array(w1977) -> (w1980:cluster{dbl[], dbl[]}[])  [unwired: 1 out]
                n988 = Array To Cluster(array=w1980) -> (cluster=w1978:T8)
                n989 = Unbundle(w1978) -> ("[0]"=w1979:cluster{dbl[], dbl[]})  [unwired: 8 out]
                n990 = Unbundle(w1979) -> (w1976:dbl[], w1975:dbl[])
                n991 = local write "Calc: STS"(w1989) -> ()
                n992 = local write "XY Graph 2"(w1977) -> ()
                n993 = local write "Index 2"(w1982) -> ()
                n994 = call "mobility_subvi_07_12a_JW.vi"("Path"=w1988, "NumPts"=w1987) -> ("Dielectric (d)"=w1992:dbl, "Index"=w1997:dbl, "XY Graph"=w2000:cluster{dbl[], dbl[]}[], "Length"=w1990:dbl, "Vt"=w1993:dbl, "Width"=w1991:dbl, "Table Control"=w2035:string[][], "Table Control 2"=w2034:string[][], "Mobility"=w2033:dbl)  [unwired: 4 in, 1 out]
                n995 = local write "Calc: VT"(w1993) -> ()
                n996 = local write "New: Dielectric"(w1992) -> ()
                n997 = Decimate 1D Array(w2000) -> (w2001:cluster{dbl[], dbl[]}[])  [unwired: 1 out]
                n998 = Array To Cluster(array=w2001) -> (cluster=w2003:T8)
                n999 = local write "Table Control"(w2035) -> ()
                n1000 = Unbundle(w2003) -> ("[0]"=w2002:cluster{dbl[], dbl[]})  [unwired: 8 out]
                n1001 = Unbundle(w2002) -> (w1984:dbl[], w1983:dbl[])
                n1002 = local write "Calc: Mobility-Sat"(w2033) -> ()
                n1003 = local write "XY Graph"(w2000) -> ()
                n1004 = local write "Table Control 2"(w2034) -> ()
                n1005 = Array Subset(array=w1984, index=w1997, length=w1987) -> (w1999:dbl[])
                n1006 = Array Subset(array=w1983, index=w1997, length=w1987) -> (w1998:dbl[])
                n1007 = local write "Array 2"(w1998) -> ()
                n1008 = local write "Array"(w1999) -> ()
                n1009 = local write "MobVi Index"(w1997) -> ()
                n1010 = local write "Slide"(w1997) -> ()
                n1011 = Array Subset(array=w1976, index=w1982, length=w1981) -> (w1986:dbl[])
                n1012 = Array Subset(array=w1975, index=w1982, length=w1981) -> (w1985:dbl[])
                n1013 = local write "New: Width"(w1991) -> ()
                n1014 = local write "Data File"(w1988) -> ()
                n1015 = local write "New: Length"(w1990) -> ()
                n1016 = local write "Folder Index"(w1961) -> ()
                n1017 = local write "Array 8"(w1986) -> ()
                n1018 = local write "Array 7"(w1985) -> ()
                n1019 = call-poly <vilib>:"Read From Spreadsheet File.vi"("file path (dialog if empty)"=w1988) -> ("all rows"=w2023:string[][])  [unwired: 6 in, 4 out]
                n1020 = local read "Image Folder"() -> (w2011:path)
                n1021 = Array Size(array=w2023) -> (size(s)=w2022:i32[])
                n1022 = List Folder(path=w2011) -> (filenames=w2016:string[])  [unwired: 3 in, 3 out]
                n1023 = Index Array(array=w2022, index=w2021) -> (element=w1995:i32)
                n1024 = Subtract(x=w1995, y=20) -> (x-y=w1994:i32)
                n1025 = property on="Slide" class="Slide (strict)"("Scale.Maximum"=w1994) -> ()  [unwired: 2 in, 2 out]
                n1026 = Array Subset(array=w2023, index (row)=w2021, index (col)=w2021, length (col)=3) -> (w2024:string[][])  [unwired: 1 in]
                n1027 = Reshape Array(w2024, w1995) -> (w2004:string[])
                n1028 = Search 1D Array(1D array=w2004, element="Mobility-Sat (cm^2/Vs):") -> (index of element=w2009:i32)  [unwired: 1 in]
                n1029 = Search 1D Array(1D array=w2004, element="Index:") -> (index of element=w2018:i32)  [unwired: 1 in]
                n1030 = Increment(x=w2018) -> (x+1=w2019:i32)
                n1031 = Index Array(array=w2004, index=w2019) -> (element=w2014:string)
                n1032 = while {
                  tunnel: w2016 -> [w2047]
                  tunnel: w2014 -> [w2045]
                  tunnel: [w2044] -> _
                  tunnel: [w2044] -> w2015
                  tunnel: w1995 -> [w2043]
                  i -> [w2044]
                  stop <- w2040 stop-if-true
                  n1033 = Index Array(array=w2047, index=w2044) -> (element=w2048:string)
                  n1034 = xnode "Match Regular Expression"("input string"=w2048, "regular expression"=w2045) -> ("whole match"=w2046:string)  [unwired: 4 in, 4 out]
                  n1035 = Equal?(x=w2046, y=w2045) -> (x = y?=w2042:bool)
                  n1036 = Equal?(x=w2043, y=w2044) -> (x = y?=w2041:bool)
                  n1037 = Or(x=w2042, y=w2041) -> (x .or. y?=w2040:bool)
                }
                n1038 = local write "Index"(w2014) -> ()
                n1039 = Increment(x=w2009) -> (x+1=w2008:i32)
                n1040 = local read "No Image"() -> (w1971:path)
                n1041 = Index Array(array=w2004, index=w2008) -> (element=w2006:string)
                n1042 = Fract/Exp String To Number(string=w2006) -> (number=w2005:dbl)  [unwired: 3 in, 1 out]
                n1043 = local write "Rec: Mobility-Sat"(w2005) -> ()
                n1044 = Path To String(path=w2011) -> (string=w2013:string)
                n1045 = local read "Image Out"() -> (w1963:T2)
                n1046 = Index Array(array=w2016, index=w2015) -> (element=w1973:string)
                n1047 = Empty String/Path?(string/path=w1973) -> (empty?=w1974:bool)
                n1048 = Concatenate Strings(w2013, "\\", w1973) -> (w2012:string)
                n1049 = local write "Image Name"(w1973) -> ()
                n1050 = String To Path(string=w2012) -> (path=w1972:path)
                n1051 = Select(t=w1971, s=w1974, f=w1972) -> (s? t:f=w1965:path)
                n1052 = local write "Image File"(w1965) -> ()
                n1053 = call "IMAQ ReadFile"("File Path"=w1965, "Image"=w1963) -> ("Image Out"=w1964:T2)  [unwired: 5 in, 4 out]
                n1054 = local write "Image Out 2"(w1964) -> ()
                n1055 = local write "Image Out"(w1964) -> ()
                n1056 = invoke on="Image Out" class="ImageControl" method="Clear ROI"() -> ()  [unwired: 3 in, 3 out]
              }
              frame #4 {
                # "Output ROI data"
                n1057 = local read "Image Folder"() -> (w2163:path)
                n1058 = Build Path(base path=w2163, name or relative path="ROI") -> (appended path=w2165:path)
                n1059 = local read "Index"() -> (w2164:string)
                n1060 = Build Path(base path=w2165, name or relative path=w2164) -> (appended path=w2170:path)
                n1061 = invoke on="Image Out" class="ImageControl" method="Clear ROI"() -> (error out=w2169:errorcluster)  [unwired: 3 in, 2 out]
                n1062 = call <vilib>:"Check if File or Folder Exists.vi"("error in (no error)"=w2169, "path"=w2170) -> ("file or folder exists?"=w2167:bool, "dup path"=w2168:path)  [unwired: 7 in, 1 out]
                n1063 = case shown="True" w2167 {
                  tunnel: w2168 -> [_ w2171]
                  frame False {
                  }
                  frame True {
                    n1064 = Read from Text File(file (use dialog)=w2171) -> (text=w2175:string)  [unwired: 3 in, 3 out]
                    n1065 = property on="Image Out" class="ImageControl"() -> ("ROI"=w2172:T9)  [unwired: 2 in, 2 out]
                    n1066 = Unflatten From String(type=w2172, binary string=w2175) -> (value=w2173:T9, error out=w2174:errorcluster)  [unwired: 3 in, 1 out]
                    n1067 = property on="Image Out" class="ImageControl"(error in=w2174, "ROI"=w2173) -> ()  [unwired: 1 in, 2 out]
                  }
                }
              }
            }
            n1068 = local write "Date Recorded"(w1805) -> ()
            n1069 = local write "Rec: Length"(w1803) -> ()
            n1070 = local write "Rec: Width"(w1802) -> ()
            n1071 = local write "Rec: Temp"(w1801) -> ()
            n1072 = flat-sequence {
              tunnel: [w1830] -> w1817
              tunnel: w1817 -> [w1844]
              frame #0 {
                # "Makes Empty File for Transformer Data"
                n1073 = local read "Data Folder"() -> (w1819:path)
                n1074 = Build Path(base path=w1819, name or relative path="Stats") -> (appended path=w1821:path)
                n1075 = call <vilib>:"Check if File or Folder Exists.vi"("path"=w1821) -> ("file or folder exists?"=w1822:bool, "dup path"=w1823:path)  [unwired: 8 in, 1 out]
                n1076 = case shown="False" w1822 {
                  tunnel: [w1827 w1829] -> w1824
                  tunnel: w1823 -> [w1828 w1829]
                  frame False {
                    n1077 = Create Folder(path (use dialog)=w1828) -> (created path=w1827:path)  [unwired: 2 in, 2 out]
                  }
                  frame True {
                  }
                }
                n1078 = Build Path(base path=w1824, name or relative path="Tranformer Data.txt") -> (appended path=w1826:path)
                n1079 = call-poly <vilib>:"Write To Spreadsheet File.vi"("append to file? (new file:F)"=TRUE, "file path (dialog if empty)"=w1826) -> ()  [unwired: 6 in, 1 out]
              }
              frame #1 {
                # "Adds Headers if they don't exist"
                n1080 = Concatenate Strings("Stats\\", "Tranformer Data.txt") -> (w1837:string)
                n1081 = local read "Data Folder"() -> (w1836:path)
                n1082 = Build Path(base path=w1836, name or relative path=w1837) -> (appended path=w1830:path)
                n1083 = call-poly <vilib>:"Read From Spreadsheet File.vi"("file path (dialog if empty)"=w1830) -> ("first row"=w1835:string[])  [unwired: 6 in, 4 out]
                n1084 = Search 1D Array(1D array=w1835, element="DeviceID") -> (index of element=w1833:i32)  [unwired: 1 in]
                n1085 = Equal?(x=w1833, y=0) -> (x = y?=w1831:bool)
                n1086 = case shown="False" w1831 {
                  tunnel: w1830 -> [w1841 _]
                  frame False {
                    n1087 = local read "Transformer \nHeaders"() -> (w1840:string[])
                    n1088 = call-poly <vilib>:"Write To Spreadsheet File.vi"("1D data"=w1840, "file path (dialog if empty)"=w1841) -> ()  [unwired: 6 in, 1 out]
                  }
                  frame True {
                  }
                }
              }
              frame #2 {
                # "Adds current device if it doesn't exist"
                n1089 = local read "Current \nRecord"() -> (w1847:string[])
                n1090 = Index Array(array=w1847, index=0) -> (element=w1846:string)
                n1091 = Concatenate Strings("Stats\\", "Tranformer Data.txt") -> (w1850:string)
                n1092 = local read "Data Folder"() -> (w1849:path)
                n1093 = local write "Current Device ID"(w1846) -> ()
                n1094 = local read "Current Device ID"() -> (w1856:string)
                n1095 = Build Path(base path=w1849, name or relative path=w1850) -> (appended path=w1848:path)
                n1096 = call-poly <vilib>:"Read From Spreadsheet File.vi"("file path (dialog if empty)"=w1848) -> ("all rows"=w1843:string[][])  [unwired: 6 in, 4 out]
                n1097 = Index Array(array=w1843, index (col)=0) -> (element=w1854:string[])  [unwired: 1 in]
                n1098 = Search 1D Array(1D array=w1854, element=w1856) -> (index of element=w1842:i32)  [unwired: 1 in]
                n1099 = Equal?(x=w1842, y=-1) -> (x = y?=w1845:bool)
                n1100 = case shown="False" w1845 {
                  tunnel: w1844 -> [w1858 w1871]
                  tunnel: w1842 -> [w1863 _]
                  tunnel: w1843 -> [w1864 _]
                  frame False {
                    n1101 = local read "Current \nRecord"() -> (w1862:string[])
                    n1102 = Replace Array Subset(array=w1864, new element=w1862, index (row)=w1863) -> (w1859:string[][])  [unwired: 1 in]
                    n1103 = flat-sequence {
                      tunnel: [w1865] -> _
                      tunnel: [w1866] -> _
                      tunnel: [w1866] -> w1861
                      tunnel: [w1865] -> w1860
                      tunnel: w1859 -> [w1866]
                      tunnel: w1858 -> [w1865]
                      tunnel: w1861 -> [w1868]
                      tunnel: w1860 -> [w1867]
                      frame #0 {
                        n1104 = Delete(path (use dialog)=w1865) -> ()  [unwired: 4 in, 3 out]
                      }
                      frame #1 {
                        n1105 = call-poly <vilib>:"Write To Spreadsheet File.vi"("append to file? (new file:F)"=TRUE, "2D data"=w1868, "file path (dialog if empty)"=w1867) -> ()  [unwired: 5 in, 1 out]
                      }
                    }
                  }
                  frame True {
                    n1106 = local read "Current \nRecord"() -> (w1870:string[])
                    n1107 = call-poly <vilib>:"Write To Spreadsheet File.vi"("append to file? (new file:F)"=TRUE, "1D data"=w1870, "file path (dialog if empty)"=w1871) -> ()  [unwired: 5 in, 1 out]
                  }
                }
              }
            }
          }
          event "Export": Mouse Down {
            n1108 = event-data() -> ()  [unwired: 1 in, 7 out]
            n1109 = call "OA_ConnectToOrigin.vi"() -> ("error out"=w2197:errorcluster, "Origin.IOApplication"=w2198:refnum<k7>)  [unwired: 8 in]
            n1110 = local read "Data Folder"() -> (w2176:path)
            n1111 = local read "Project"() -> (w2196:path)
            n1112 = call "OA_Load.vi"("error in (no error)"=w2197, "Path"=w2196, "Origin.IOApplication"=w2198) -> ("error out"=w2189:errorcluster, "Origin.IOApplication"=w2190:refnum<k7>)  [unwired: 1 out]
            n1113 = call "OAExecute.vi"("script"="document -m 3;", "Error IO"=w2189, "Origin.IOApplication"=w2190) -> ("Error IO Out"=w2187:errorcluster, "Origin.IOApplication"=w2188:refnum<k7>)  [unwired: 1 in, 1 out]
            n1114 = Build Path(base path=w2176, name or relative path="Stats") -> (appended path=w2177:path)
            n1115 = flat-sequence {
              tunnel: w2176 -> [w2218]
              tunnel: w2195 -> [w2217]
              tunnel: [w2207] -> w2200
              tunnel: [w2208] -> w2199
              tunnel: w2188 -> [w2212]
              tunnel: w2187 -> [w2211]
              tunnel: w2176 -> [w2234]
              tunnel: w2195 -> [w2233]
              tunnel: w2200 -> [w2229]
              tunnel: w2199 -> [w2230]
              tunnel: [w2224] -> w2194
              tunnel: [w2223] -> w2193
              tunnel: w2176 -> [w2245]
              tunnel: w2195 -> [w2244]
              tunnel: w2194 -> [w2240]
              tunnel: w2193 -> [w2239]
              tunnel: [w2238] -> w2192
              tunnel: [w2237] -> w2191
              tunnel: w2176 -> [w2260]
              tunnel: w2195 -> [w2259]
              tunnel: w2192 -> [w2254]
              tunnel: w2191 -> [w2253]
              tunnel: [w2251] -> w2185
              tunnel: [w2250] -> w2184
              frame #0 {
                n1116 = call "Param_Analysis.vi"("error in (no error)"=w2211, "Folder 2"=w2218, "Parameter String"="Mobility (cm^2/Vs):", "Parameter Name"="Mobility", "Folder"=w2217) -> ("error out"=w2214:errorcluster, "Array 4"=w2204:string[], "Array 3"=w2213:string[][])  [unwired: 3 in, 1 out]
                n1117 = call "Origin_Export.vi"("String 3"="[MobHistTab]Sheet1", "error in (no error)"=w2214, "Array"=w2213, "String 2"="[MOBvsLTable]Mobilities", "String"="pe_cd \"Mobility Chart\";", "Origin.IOApplication"=w2212, "Array 2"=w2204) -> ("reference out"=w2210:refnum<k7>, "error out"=w2209:errorcluster)  [unwired: 2 in, 1 out]
                n1118 = call "OAExecute.vi"("script"="window -a MOBvsLTable;\nwindow -s TV;", "Error IO"=w2209, "Origin.IOApplication"=w2210) -> ("Error IO Out"=w2207:errorcluster, "Origin.IOApplication"=w2208:refnum<k7>)  [unwired: 1 in, 1 out]
              }
              frame #1 {
                n1119 = call "Param_Analysis.vi"("error in (no error)"=w2229, "Folder 2"=w2234, "Parameter String"="On/Off Current:", "Parameter Name"="On_Off_Current", "Folder"=w2233) -> ("error out"=w2228:errorcluster, "Array 4"=w2222:string[], "Array 3"=w2225:string[][])  [unwired: 3 in, 1 out]
                n1120 = call "Origin_Export.vi"("String 3"="[OnOffHistTab]Sheet1", "error in (no error)"=w2228, "Array"=w2225, "String 2"="[OnOffTable]On/Off Ratios", "String"="pe_cd \"OnOff vs L\";", "Origin.IOApplication"=w2230, "Array 2"=w2222) -> ("reference out"=w2224:refnum<k7>, "error out"=w2223:errorcluster)  [unwired: 2 in, 1 out]
              }
              frame #2 {
                n1121 = call "Param_Analysis.vi"("Folder 2"=w2245, "Parameter String"="S.T.S. (V/decade):", "Parameter Name"="STS", "Folder"=w2244) -> ("Array 4"=w2236:string[], "Array 3"=w2241:string[][])  [unwired: 4 in, 2 out]
                n1122 = call "Origin_Export.vi"("String 3"="[SHistTab]Sheet1", "error in (no error)"=w2239, "Array"=w2241, "String 2"="[STable]Threshold Swing", "String"="pe_cd \"Threshold Swing vs L\";", "Origin.IOApplication"=w2240, "Array 2"=w2236) -> ("reference out"=w2237:refnum<k7>, "error out"=w2238:errorcluster)  [unwired: 2 in, 1 out]
              }
              frame #3 {
                n1123 = call "Param_Analysis.vi"("Folder 2"=w2260, "Parameter String"="Threshold V (V):", "Parameter Name"="Threshold_V", "Folder"=w2259) -> ("Array 4"=w2249:string[], "Array 3"=w2252:string[][])  [unwired: 4 in, 2 out]
                n1124 = call "Origin_Export.vi"("String 3"="[VtHistTab]Sheet1", "error in (no error)"=w2254, "Array"=w2252, "String 2"="[VtTable]Threshold Voltages", "String"="pe_cd \"Threshold Voltage vs L\";", "Origin.IOApplication"=w2253, "Array 2"=w2249) -> ("reference out"=w2251:refnum<k7>, "error out"=w2250:errorcluster)  [unwired: 2 in, 1 out]
              }
            }
            n1125 = call <vilib>:"Check if File or Folder Exists.vi"("path"=w2177) -> ("file or folder exists?"=w2202:bool, "dup path"=w2201:path)  [unwired: 8 in, 1 out]
            n1126 = case shown="False" w2202 {
              tunnel: w2201 -> [w2262 w2263]
              tunnel: [w2261 w2263] -> w2195
              frame False {
                n1127 = Create Folder(path (use dialog)=w2262) -> (created path=w2261:path)  [unwired: 2 in, 2 out]
              }
              frame True {
              }
            }
            n1128 = call "File Dialog"("start path"=w2177) -> ("selected path"=w2180:path)  [unwired: 11 in, 3 out]
            n1129 = Path To String(path=w2180) -> (string=w2179:string)
            n1130 = call "OAExecute.vi"("script"="pe_cd /;\npe_cd \"Mobility Chart\"; ", "Error IO"=w2184, "Origin.IOApplication"=w2185) -> ("Error IO Out"=w2181:errorcluster, "Origin.IOApplication"=w2182:refnum<k7>)  [unwired: 1 in, 1 out]
            n1131 = call "OASaveProject.vi"("path"=w2179, "Error IO"=w2181, "Origin.IOApplication"=w2182) -> ()  [unwired: 3 out]
          }
          event "Blank Button": Mouse Down {
            n1132 = event-data() -> ()  [unwired: 1 in, 7 out]
            n1133 = local read "Data File"() -> (w2271:path)
            n1134 = Strip Path(path=w2271) -> (stripped path=w2267:path, name=w2269:string)
            n1135 = Path To String(path=w2267) -> (string=w2266:string)
            n1136 = Concatenate Strings(w2266, "\\", "X_", w2269) -> (w2265:string)
            n1137 = String To Path(string=w2265) -> (path=w2264:path)
            n1138 = Move(source path=w2271, 10:w2264) -> ()  [unwired: 3 in, 3 out]
            n1139 = local write "Data File"(w2264) -> ()
          }
          event "Cancel Button": Mouse Down {
            (unwired) 6
            n1140 = event-data() -> ()  [unwired: 1 in, 7 out]
            n1141 = call "Simulate_Keyboard.vi"("Action"=2, "Virtual Key"=162) -> ()  [unwired: 7 in, 1 out]
          }
        }
        n1142 = Reciprocal(x=w487) -> (1/x=w486:sgl)
        n1143 = Multiply(x=w486, y=10) -> (x*y=w488:sgl)
        n1144 = case shown="\"EQUALS\"" w527 {
          tunnel: w501 -> [w576 w582 w586 w588 w592 w594 w596 w598 w600 w602 w604 w606 w608 w610 w612 w614 w616 w618 w620 w622 w624 w626 w628 w630 w632 w634 w636 w638 w640 w642 w644 w646 w648 w650 w652 w654 w656 w658 w660 w662 w664 w666 w668 w670 w672 w674 w676 w678 w680 w682 w684 w686 w688 w690 w692 w694 w696 w698 w700 w702 w704 w706 w708 w710 w712 w714 w716 w718 w720 w722 w724 w726 w728 w730 w732 w734 w736 w738 w740 w742 w744 w746 w748 w750 w752 w754 w756 w758 w760 w762 w764 w766 w768 w770 w772 w774 w776 w778 w780 w782 w784 w786 w788 w790 w792]
          tunnel: [w576 w581 w585 w588 w592 w594 w596 w598 w600 w602 w604 w606 w608 w610 w612 w614 w616 w618 w620 w622 w624 w626 w628 w630 w632 w634 w636 w638 w640 w642 w644 w646 w648 w650 w652 w654 w656 w658 w660 w662 w664 w666 w668 w670 w672 w674 w676 w678 w680 w682 w684 w686 w688 w690 w692 w694 w696 w698 w700 w702 w704 w706 w708 w710 w712 w714 w716 w718 w720 w722 w724 w726 w728 w730 w732 w734 w736 w738 w740 w742 w744 w746 w748 w750 w752 w754 w756 w758 w760 w762 w764 w766 w768 w770 w772 w774 w776 w778 w780 w782 w784 w786 w788 w790 w792] -> w526
          tunnel: w502 -> [w578 w580 w584 w590 w591 w593 w595 w597 w599 w601 w603 w605 w607 w609 w611 w613 w615 w617 w619 w621 w623 w625 w627 w629 w631 w633 w635 w637 w639 w641 w643 w645 w647 w649 w651 w653 w655 w657 w659 w661 w663 w665 w667 w669 w671 w673 w675 w677 w679 w681 w683 w685 w687 w689 w691 w693 w695 w697 w699 w701 w703 w705 w707 w709 w711 w713 w715 w717 w719 w721 w723 w725 w727 w729 w731 w733 w735 w737 w739 w741 w743 w745 w747 w749 w751 w753 w755 w757 w759 w761 w763 w765 w767 w769 w771 w773 w775 w777 w779 w781 w783 w785 w787 w789 w791]
          tunnel: [w577 w580 w584 w589 w591 w593 w595 w597 w599 w601 w603 w605 w607 w609 w611 w613 w615 w617 w619 w621 w623 w625 w627 w629 w631 w633 w635 w637 w639 w641 w643 w645 w647 w649 w651 w653 w655 w657 w659 w661 w663 w665 w667 w669 w671 w673 w675 w677 w679 w681 w683 w685 w687 w689 w691 w693 w695 w697 w699 w701 w703 w705 w707 w709 w711 w713 w715 w717 w719 w721 w723 w725 w727 w729 w731 w733 w735 w737 w739 w741 w743 w745 w747 w749 w751 w753 w755 w757 w759 w761 w763 w765 w767 w769 w771 w773 w775 w777 w779 w781 w783 w785 w787 w789 w791] -> w525
          tunnel: w488 -> [w575 w579 w583 w587 _ _ _ _ _ _ _ _ _ _ _ _ _ _ _ _ _ _ _ _ _ _ _ _ _ _ _ _ _ _ _ _ _ _ _ _ _ _ _ _ _ _ _ _ _ _ _ _ _ _ _ _ _ _ _ _ _ _ _ _ _ _ _ _ _ _ _ _ _ _ _ _ _ _ _ _ _ _ _ _ _ _ _ _ _ _ _ _ _ _ _ _ _ _ _ _ _ _ _ _ _]
          frame "DOWN" {
            n1145 = Add(x=w578, y=w575) -> (x+y=w577:sgl)
          }
          frame "LEFT" {
            n1146 = Subtract(x=w582, y=w579) -> (x-y=w581:sgl)
          }
          frame "RIGHT" {
            n1147 = Add(x=w586, y=w583) -> (x+y=w585:sgl)
          }
          frame "UP" {
            n1148 = Subtract(x=w590, y=w587) -> (x-y=w589:sgl)
          }
          frame "ENTER (num pad)" {
          }
          frame "' (quote)" {
          }
          frame "END" {
          }
          frame "EQUALS" {
          }
          frame "ESCAPE" {
          }
          frame "GRAVE (`)" {
          }
          frame "HOME" {
          }
          frame "INSERT" {
          }
          frame "LBRACKET" {
          }
          frame "LCONTROL" {
          }
          frame "L ALT" {
          }
          frame "LSHIFT" {
          }
          frame "LWIN" {
          }
          frame "MINUS" {
          }
          frame "MULTIPLY" {
          }
          frame "NEXT" {
          }
          frame "NUMLOCK" {
          }
          frame "NUMPAD_0" {
          }
          frame "NUMPAD_1" {
          }
          frame "NUMPAD_2" {
          }
          frame "NUMPAD_3" {
          }
          frame "NUMPAD_4" {
          }
          frame "NUMPAD_5" {
          }
          frame "NUMPAD_6" {
          }
          frame "NUMPAD_7" {
          }
          frame "NUMPAD_8" {
          }
          frame "NUMPAD_9" {
          }
          frame "PAUSE" {
          }
          frame "PERIOD" {
          }
          frame "PRIOR (PG UP)" {
          }
          frame "RBRACKET" {
          }
          frame "RCONTROL" {
          }
          frame "RETURN" {
          }
          frame "R ALT" {
          }
          frame "RSHIFT" {
          }
          frame "RWIN" {
          }
          frame "SCROLL" {
          }
          frame "SEMICOLON" {
          }
          frame "SLASH" {
          }
          frame "SPACE" {
          }
          frame "SUBTRACT" {
          }
          frame "TAB" {
          }
          frame "DIVIDE" {
          }
          frame "DELETE" {
          }
          frame "DECIMAL" {
          }
          frame "COMMA" {
          }
          frame "CAPITAL" {
          }
          frame "BACKSLASH" {
          }
          frame "BACK" {
          }
          frame "ADD" {
          }
          frame "F15" {
          }
          frame "F14" {
          }
          frame "F13" {
          }
          frame "F12" {
          }
          frame "F11" {
          }
          frame "F10" {
          }
          frame "F9" {
          }
          frame "F8" {
          }
          frame "F7" {
          }
          frame "F6" {
          }
          frame "F5" {
          }
          frame "F4" {
          }
          frame "F3" {
          }
          frame "F2" {
          }
          frame "F1" {
          }
          frame "Z" {
          }
          frame "Y" {
          }
          frame "X" {
          }
          frame "W" {
          }
          frame "V" {
          }
          frame "U" {
          }
          frame "T" {
          }
          frame "S" {
          }
          frame "R" {
          }
          frame "Q" {
          }
          frame "P" {
          }
          frame "O" {
          }
          frame "N" {
          }
          frame "M" {
          }
          frame "L" {
          }
          frame "K" {
          }
          frame "J" {
          }
          frame "I" {
          }
          frame "H" {
          }
          frame "G" {
          }
          frame "F" {
          }
          frame "E" {
          }
          frame "D" {
          }
          frame "C" {
          }
          frame "B" {
          }
          frame "A" {
          }
          frame "9" {
          }
          frame "8" {
          }
          frame "7" {
          }
          frame "6" {
          }
          frame "5" {
          }
          frame "4" {
          }
          frame "3" {
          }
          frame "2" {
          }
          frame "1" {
          }
          frame "0" {
          }
        }
        n1149 = Bundle(w504, w503, w518, w517, 0.0) -> (w516:cluster{dbl, dbl, dbl, dbl, dbl})  [unwired: 1 in]
        n1150 = Bundle("X"=w526, "Y"=w525) -> (w520:cluster{"X":sgl, "Y":sgl})  [unwired: 1 in]
        n1151 = Divide(x=20, y=w487) -> (x/y=w490:sgl)
        n1152 = property on="Image Out" class="ImageControl"("Image Center Position"=w520) -> ()  [unwired: 2 in, 2 out]
        n1153 = call "IMAQ Convert Rectangle to ROI (Polygon)"("Rectangle"=w516) -> ("ROI Descriptor"=w514:T3)  [unwired: 7 in, 2 out]
        n1154 = Bundle("Application Font", w490, w494, w494, w494, w494, w494, TRUE, w492) -> (w496:T15)  [unwired: 1 in]
        n1155 = property on="Image Out 2" class="ImageControl"("ROI"=w514) -> ()  [unwired: 2 in, 2 out]
        n1156 = Bundle(w492, w496, w492, w492) -> (w495:T16)  [unwired: 1 in]
        n1157 = property on="Image Out" class="ImageControl"() -> ("ROI"=w469:T9)  [unwired: 2 in, 2 out]
        n1158 = Unbundle By Name(w469) -> ("Contours"=w543:T12)
        n1159 = local read "Image Out"() -> (w498:T2)
        n1160 = call "IMAQ Clear Overlay"("Image"=w498) -> ("Image Out"=w497:T2)  [unwired: 9 in, 1 out]
        n1161 = Initialize Array(0) -> (w541:i32[])  [unwired: 1 in]
        n1162 = local read "Magnification"() -> (w532:u16)
        n1163 = Array Size(array=w543) -> (size(s)=w542:i32)
        n1164 = Build Array(0.505025, 0.252522, 0.127742, 0.050345, 0.031129) -> (w533:dbl[])
        n1165 = Array Subset(array=w533, index=w532, length=1) -> (w530:dbl[])
        n1166 = property on="Image Out" class="ImageControl"() -> ("ZoomInteger"=w522:cluster{"X":i32, "Y":i32})  [unwired: 2 in, 2 out]
        n1167 = To Double Precision Float(number=w530) -> (double precision float=w529:dbl[])
        n1168 = for {
          N: w542 -> [_]
          shift-right: [w815] -> _
          shift-left: w543 -> [w815]
          shift-right: [w813] -> w528
          shift-left: w541 -> [w812]
          tunnel: w529 -> [w811]
          shift-right: [w808] -> _
          shift-left: w497 -> [w810]
          tunnel: w495 -> [w803]
          i -> [w807]
          n1169 = Index Array(array=w815, index=w807) -> (element=w824:T17)
          n1170 = Unbundle(w824) -> ("Points"=w823:i32[])  [unwired: 2 out]
          n1171 = Array To Cluster(array=w823) -> (cluster=w822:T18)
          n1172 = Unbundle(w822) -> ("Points[0]"=w802:i32, "Points[1]"=w799:i32, "Points[2]"=w814:i32, "Points[3]"=w820:i32)  [unwired: 5 out]
          n1173 = Add(x=w802, y=10) -> (x+y=w800:i32)
          n1174 = Subtract(x=w799, y=w820) -> (x-y=w819:i32)
          n1175 = Subtract(x=w802, y=w814) -> (x-y=w821:i32)
          n1176 = Square(x=w819) -> (x^2=w817:i32)
          n1177 = Square(x=w821) -> (x^2=w818:i32)
          n1178 = Add(x=w818, y=w817) -> (x+y=w816:i32)
          n1179 = Square Root(x=w816) -> (sqrt(x)=w793:dbl)
          n1180 = Multiply(x=w793, y=0.5) -> (x*y=w796:dbl)
          n1181 = Add(x=w796, y=w799) -> (x+y=w798:dbl)
          n1182 = Bundle(w800, w798) -> (w809:cluster{i32, dbl})  [unwired: 1 in]
          n1183 = Multiply(x=w793, y=w811) -> (x*y=w806:dbl[])
          n1184 = Index Array(array=w806) -> (element=w805:dbl)  [unwired: 1 in]
          n1185 = Number To Fractional String(number=w805) -> (F-format string=w804:string)  [unwired: 3 in]
          n1186 = call "IMAQ Overlay Text"("BG Color (Transparent)"=u32 0, "Text Color (black)"=u32 16448250, "Font, Size & Style"=w803, "String"=w804, "Origin"=w809, "Image"=w810) -> ("Image Out"=w808:T2)  [unwired: 4 in, 1 out]
          n1187 = Build Array (concatenate)(w812, w806) -> (w813:dbl[])
          n1188 = local write "Numeric 3"(w793) -> ()
        }
        n1189 = local write "ROI Descriptor"(w469) -> ()
        n1190 = Unbundle(w522) -> ("X"=w521:i32)  [unwired: 1 out]
        n1191 = Add Array Elements(numeric array=w528) -> (sum=w539:dbl)
        n1192 = local write "Distances"(w528) -> ()
        n1193 = local write "Total Width"(w539) -> ()
        n1194 = local write "Zoom"(w521) -> ()
        n1195 = local read "Rec: Width"() -> (w470:dbl)
        n1196 = local read "Manual"() -> (w468:bool)
        n1197 = Not(x=w468) -> (.not. x?=w466:bool)
        n1198 = local read "Total Width"() -> (w472:dbl)
        n1199 = Equal To 0?(x=w472) -> (x = 0?=w467:bool)
        n1200 = And(x=w467, y=w466) -> (x .and. y?=w465:bool)
        n1201 = case shown="True" w465 {
          tunnel: w470 -> [_ w553]
          frame False {
          }
          frame True {
            n1202 = local write "New: Width"(w553) -> ()
          }
        }
        n1203 = Or(x=w467, y=w468) -> (x .or. y?=w471:bool)
        n1204 = case shown="False" w471 {
          tunnel: w472 -> [w554 _]
          frame False {
            n1205 = local write "New: Width"(w554) -> ()
          }
          frame True {
          }
        }
      }
    }
  }
  n1206 = Build Array("DeviceID", "Fabricator", "Deposition", "Date", "Sample", "Row", "Column", "L (um)", "W (um)", "Material", "Treatment", "TC (mM)", "Solvent", "C (%)", "ST (C)", "Drops", "Wait (s)", "RT (F)", "RH (%)", "Ramp (s)", "RPM", "Accel (RPM/s)", "Time (s)", "Mobility", "On/Off", "Vt", "S.T.S") -> (→"Transformer \nHeaders":string[])
